vi "cursor window logic V3.vi"(4 "h. offset":dbl, 6 "CursIdx":i32, 7 "cursor window action":T3=enum."check", 8 "window":dbl=nan, 9 "center":dbl=nan, 10 "cursor window in":refnum<vi>, 11 "cursor window init":T2={"left"=2378.60310421286, "right "=2421.6740576496672, "center"=2421.6740576496672, "window"=2421.6740576496672, "cursors"=[], "relative"=0, "absolute"=0, "fixed vertical offset"=2421.6740576496672, "vertical offset"=2421.6740576496672, "skew"=2421.6740576496672, "default window frac"=2421.6740576496672, "kind"=enum."skewed", "skew.left"=2421.6740576496672, "skew.right"=2421.6740576496672, "Plot ref"=refnum, "wing order"=enum."back"}) -> (2 "cursor window out":refnum<vi>, 3 "cursor window out":T2={"left"=2378.60310421286, "right "=2421.6740576496672, "center"=2421.6740576496672, "window"=2421.6740576496672, "cursors"=[], "relative"=0, "absolute"=0, "fixed vertical offset"=2421.6740576496672, "vertical offset"=2421.6740576496672, "skew"=2421.6740576496672, "default window frac"=2421.6740576496672, "kind"=enum."skewed", "skew.left"=2421.6740576496672, "skew.right"=2421.6740576496672, "Plot ref"=refnum, "wing order"=enum."back"})   [LabVIEW 2020]
uses:
  cursor window action.ctl
  cursor winow.ctl
  comparison control.ctl
  cursor window state.ctl
  stack action -- control.ctl
  cursor action.ctl
  2Dwindow.ctl
  range multiplier action.ctl
  cursor sate.ctl
  Q - not nan -- real.vi
  Q - not nan -- integer.vi
panel:
  out "selector":T1
  out "result":bool
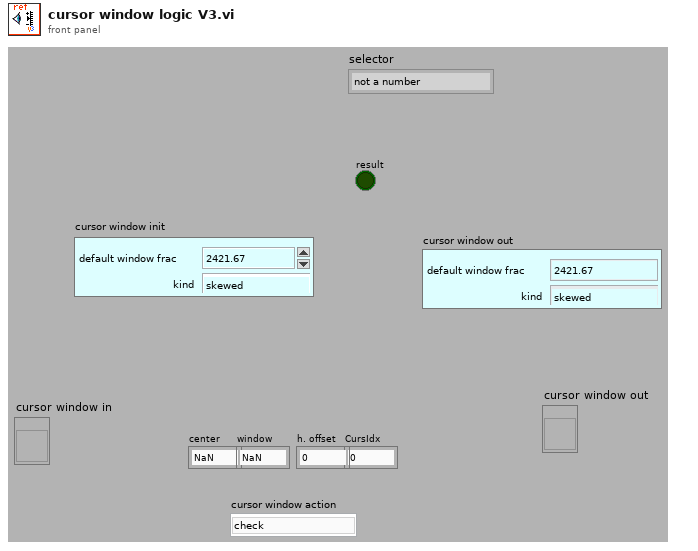
[diagram p1: front panel]
types:
  T1 = typedef "comparison control.ctl" = enum16{"not a number", "above", "in range", "below"}
  T2 = typedef "cursor winow.ctl" = cluster{"left":dbl, "right ":dbl, "center":dbl, "window":dbl, "cursors":i32[], "relative":i32, "absolute":i32, "fixed vertical offset":dbl, "vertical offset":dbl, "skew":dbl, "default window frac":dbl, "kind":enum16{"symmetric", "skewed", "fancy"}, "skew.left":dbl, "skew.right":dbl, "Plot ref":refnum<vi>, "wing order":enum16{"forw", "back"}}
  T3 = typedef "cursor window action.ctl" = enum16{"balance", "h. offset change", "cursor moves", "change center", "change window", "init", "check", "reset", "set y to middle", "idle", "-write all Y", "-write left.X", "-write center.X", "-write right.X", "-write all X", "-change center", "-change window", "-change skew", "-read cursor 2", "-read cursor 1", "-read cursor 0", "-read all cursors", "-reset", "-read plot scale", "-set y to middle", "-Q: center.Y is visible", "-Q: window is visible", "-parse center.Y", "-right left from center", "-left move", "-right move", "-set center.Y", "-empty", "-set cursors to default", "-check", "-write center.Y", "-copy cursor 1", "-copy cursor 0", "-copy cursor 2", "move right", "move left", "shrink", "broaden", "skew up", "skew down", "-write plot scale", "zoom X", "change cen&win", "zoom to all data", "color--red", "color--green", "color--yellow", "read", "zoom out", "zoom in", "slide right", "slide left", "set range aspect ratio to 1"}
  T4 = typedef "cursor window state.ctl" = cluster{"right.Y":dbl, "right.X":dbl, "left.X":dbl, "left.Y":dbl, "center.X":dbl, "center.Y":dbl, "scale.x.max":dbl, "scale.x.min":dbl, "scale.y.range":dbl, "scale.y.min":dbl, "scale.x.range":dbl, "scale.y.max":dbl, "skew":dbl, "cursor":i32, "scale.x.center":dbl, "scale.x.halfwidth":dbl, "scale.y.center":dbl, "scale.y.halfwidth":dbl}
  T5 = typedef "stack action -- control.ctl" = enum16{"push", "pop", "check", "init"}
  T6 = cluster{"center":dbl, "window":dbl, "h.offset":dbl, "cursor window":T2}
  T7 = cluster{"right.Y":dbl, "right.X":dbl, "left.X":dbl, "left.Y":dbl, "center.X":dbl, "center.Y":dbl, "scale.x.max":dbl, "scale.x.min":dbl, "scale.y.range":dbl, "scale.y.min":dbl, "scale.x.range":dbl, "scale.y.max":dbl, "skew":dbl, "cursor":i32, "scale.x.center":dbl, "scale.x.halfwidth":dbl, "scale.y.center":dbl, "scale.y.halfwidth":dbl}
  T8 = cluster{"left":dbl, "right ":dbl, "center":dbl, "window":dbl, "cursors":i32[], "relative":i32, "absolute":i32, "fixed vertical offset":dbl, "vertical offset":dbl, "skew":dbl, "default window frac":dbl, "kind":enum16{"symmetric", "skewed", "fancy"}, "skew.left":dbl, "skew.right":dbl, "Plot ref":refnum<vi>, "wing order":enum16{"forw", "back"}}
  T9 = typedef "cursor action.ctl" = enum16{"range", "read", "write", "check", "zoom out", "smart zoom out", "zoom to aspect ratio 1", "zoom to win", "zoom out 20%", "zoom in 20%", "-empty", "smart zoom out&aspect", "move range left 20%", "move range right 20%", "move range up 20%", "move range down 20%", "zoom to X win", "zoom to Y win", "zoom out X", "zoom out Y", "zoom in X", "zoom in Y", "check plot scale"}
  T10 = typedef "2Dwindow.ctl" = cluster{"window y":dbl, "center x":dbl, "center y":dbl, "window x":dbl}
  T11 = typedef "range multiplier action.ctl" = enum16{"shift", "zoom", "check"}
  T12 = typedef "2Dwindow-bounds.ctl" = cluster{"min y":dbl, "max x":dbl, "min x":dbl, "max y":dbl}
  T13 = typedef "cursor sate.ctl" = enum16{"normal", "alert", "fuzzy", "interesting", "boring", "colored"}
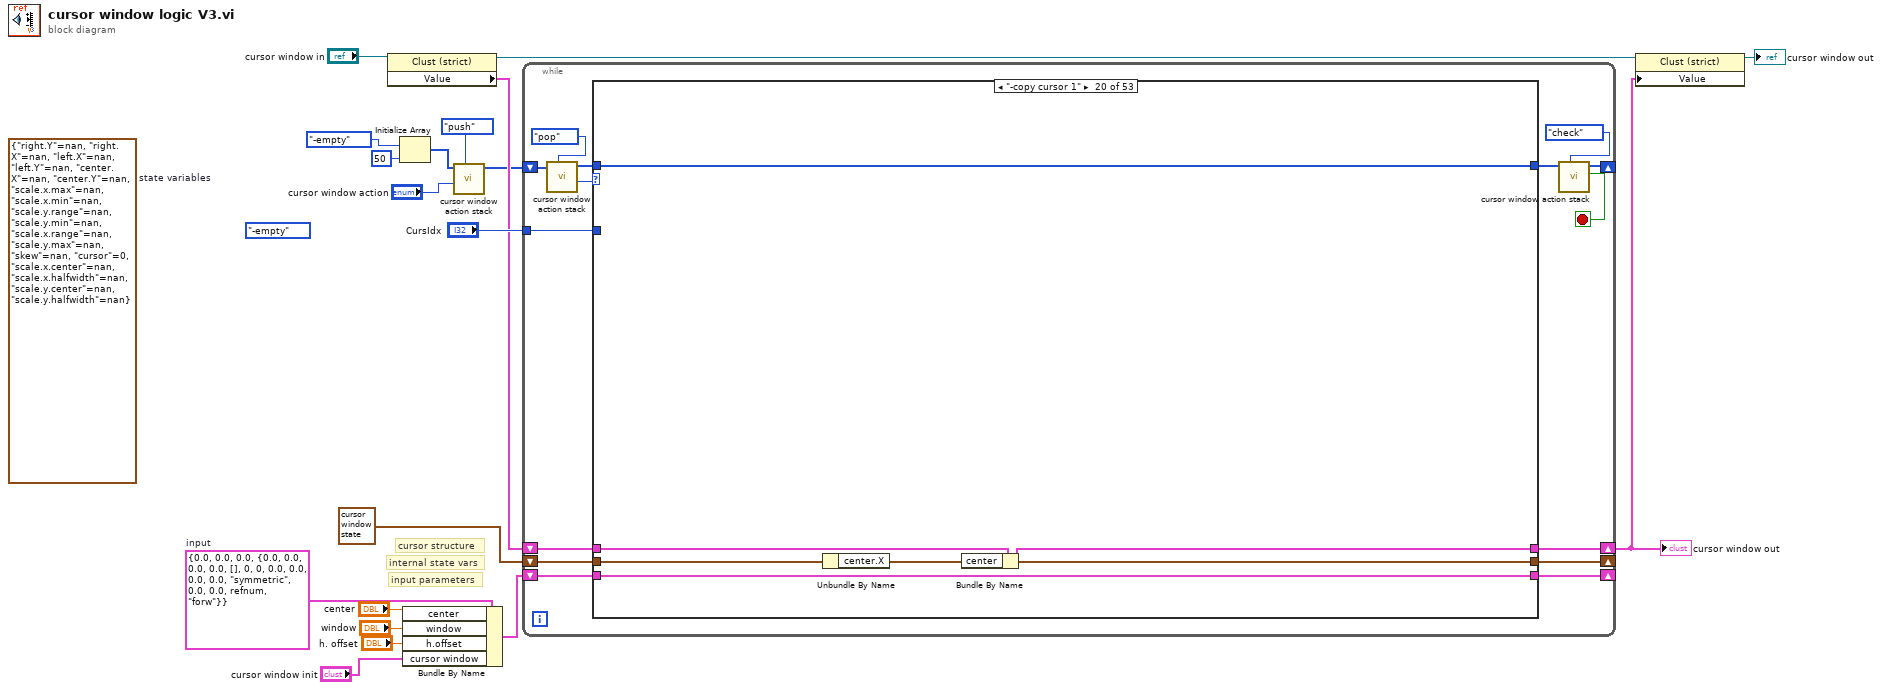
[diagram p0: block diagram]
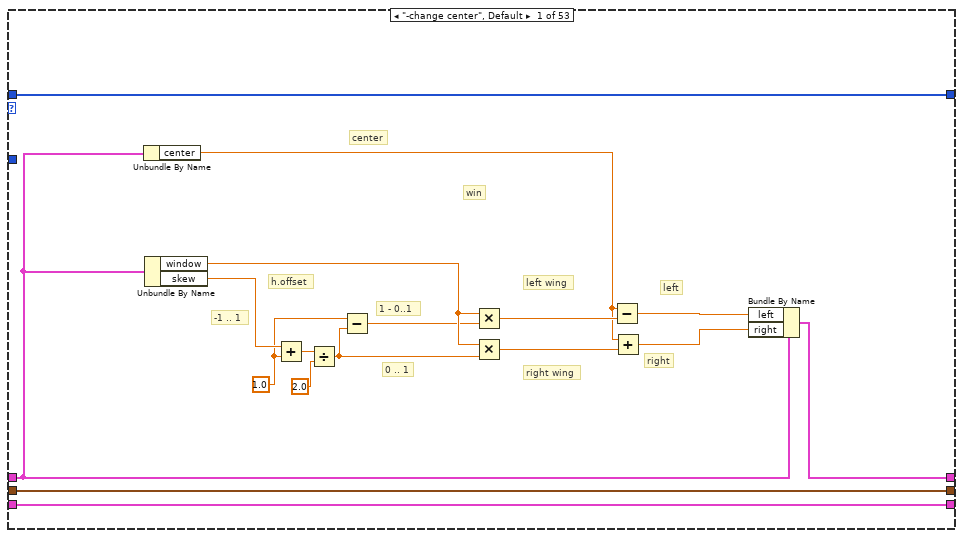
[diagram p2: hidden frame]
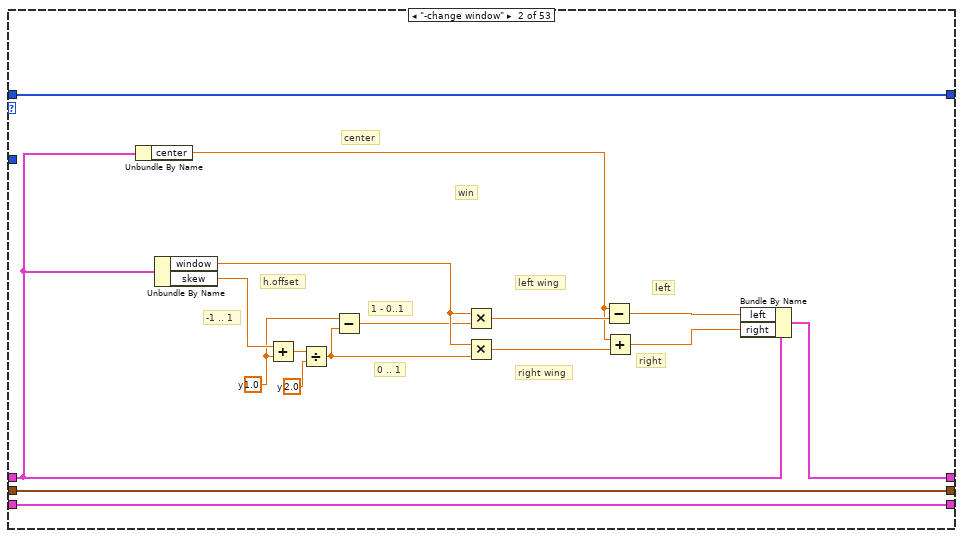
[diagram p3: hidden frame]
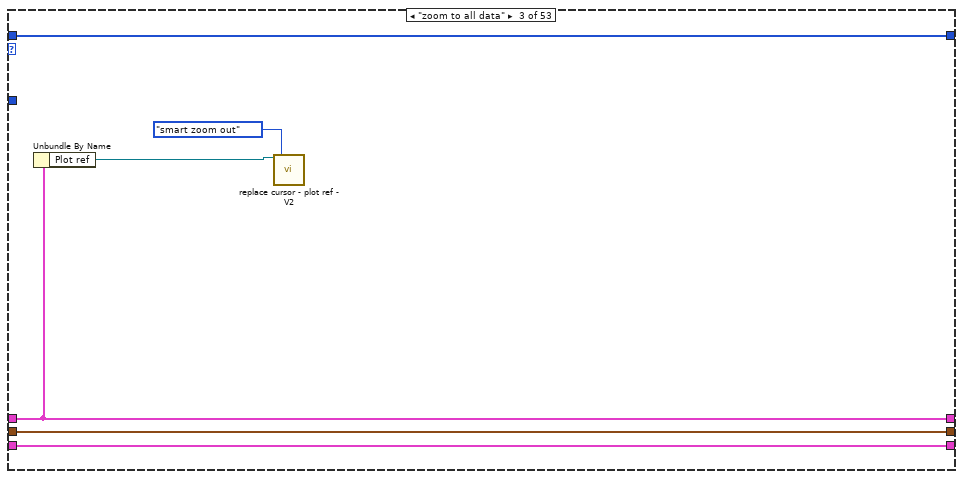
[diagram p4: hidden frame]
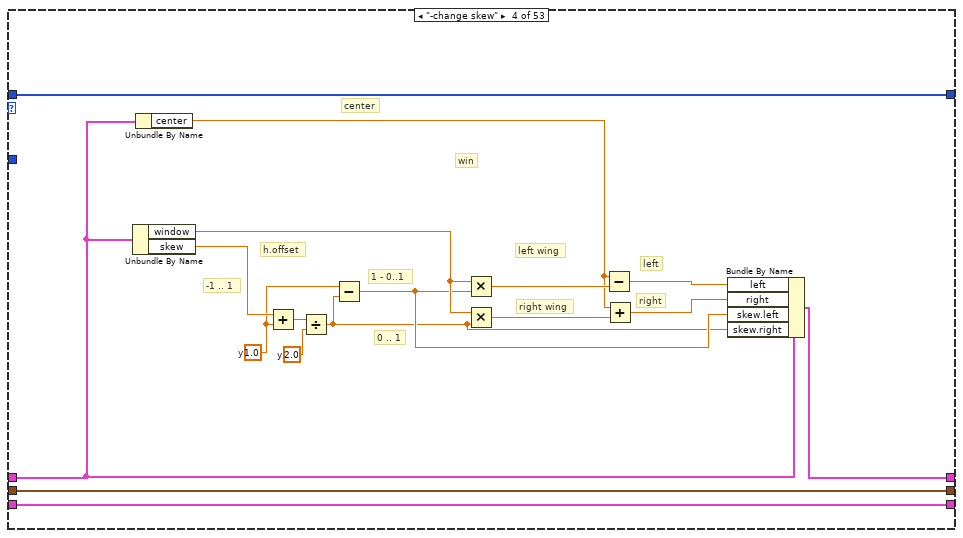
[diagram p5: hidden frame]
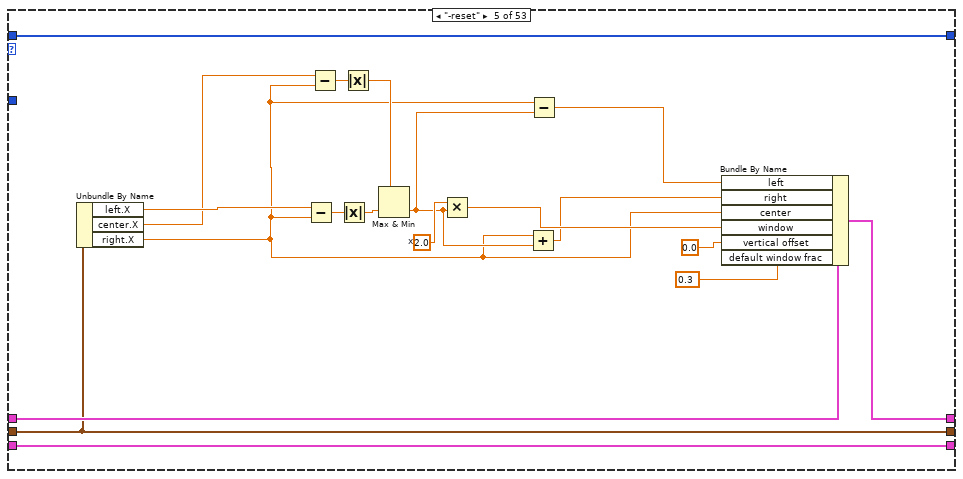
[diagram p6: hidden frame]
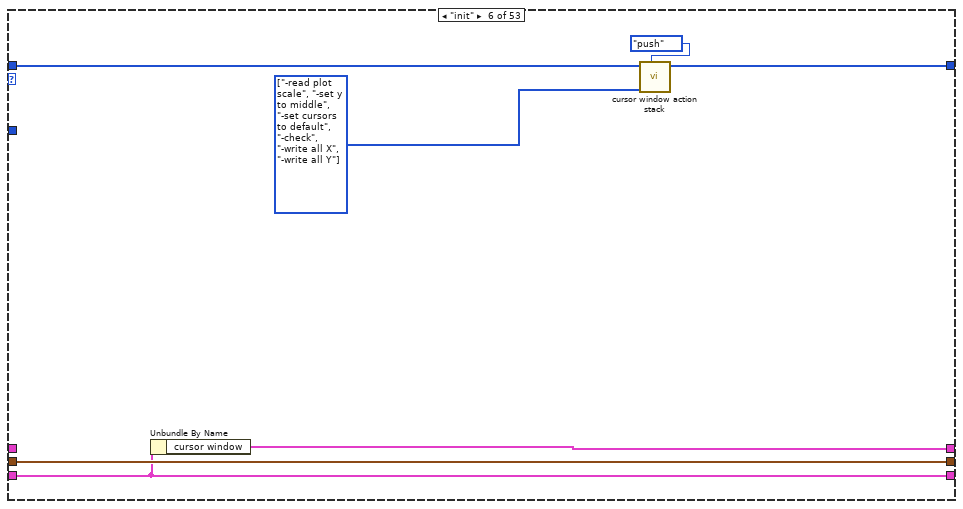
[diagram p7: hidden frame]
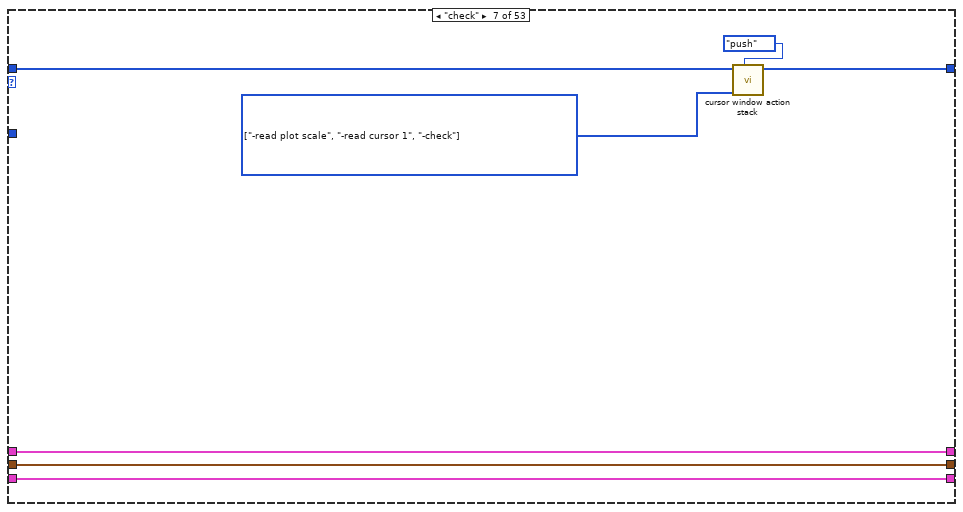
[diagram p8: hidden frame]
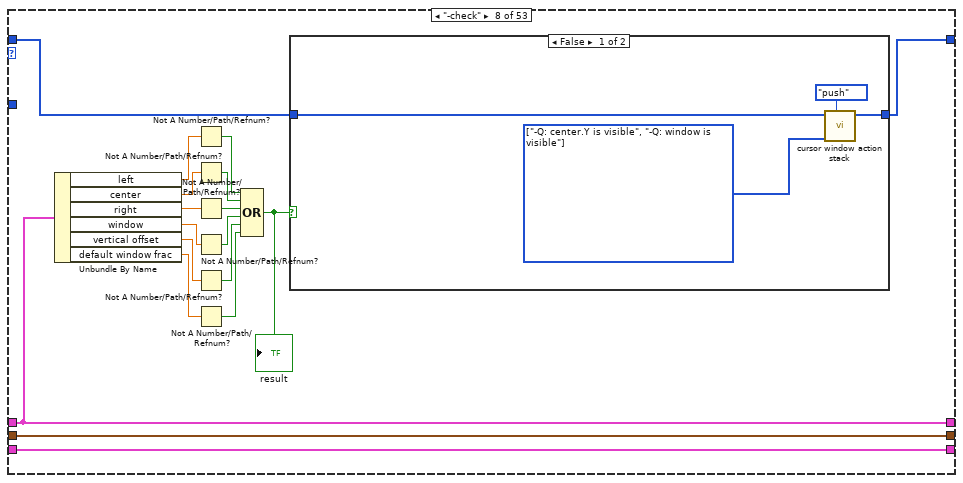
[diagram p9: hidden frame]
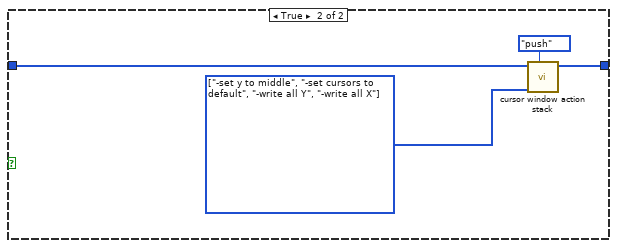
[diagram p10: hidden frame]
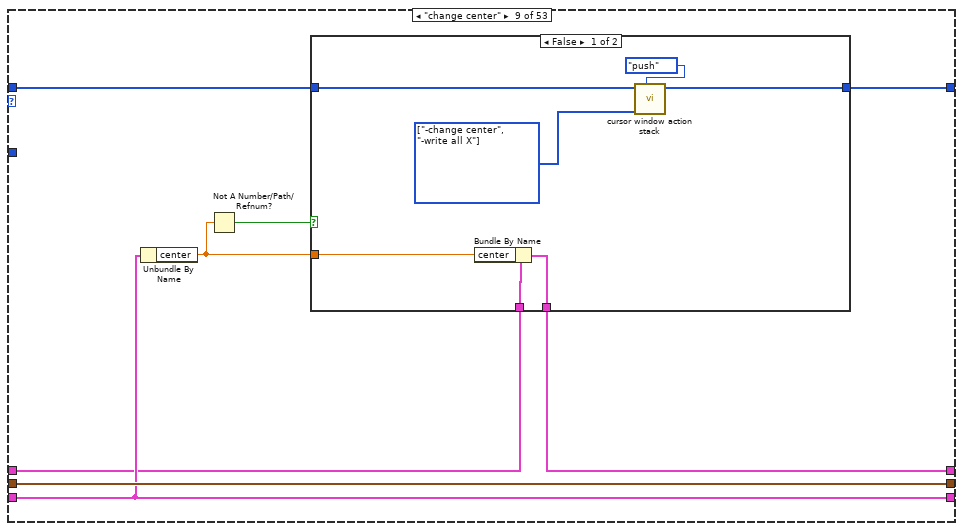
[diagram p11: hidden frame]
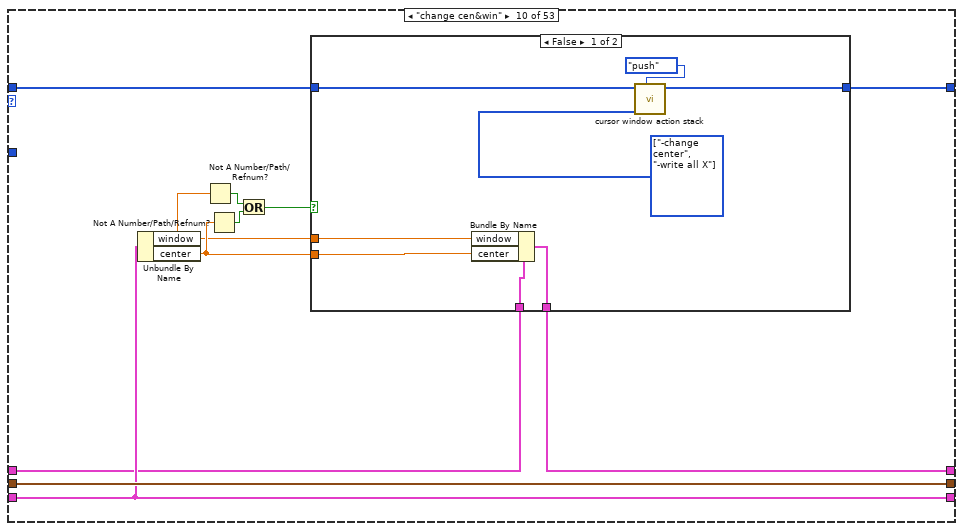
[diagram p13: hidden frame]
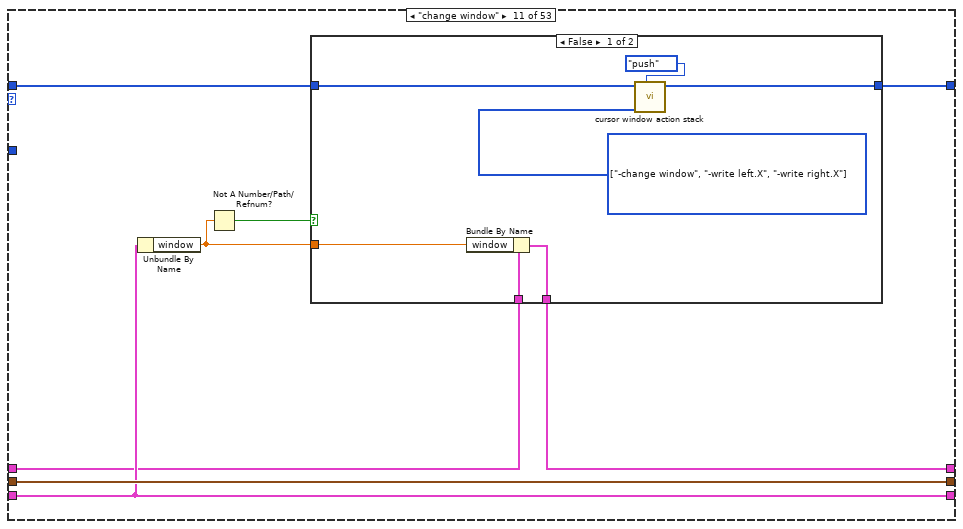
[diagram p15: hidden frame]
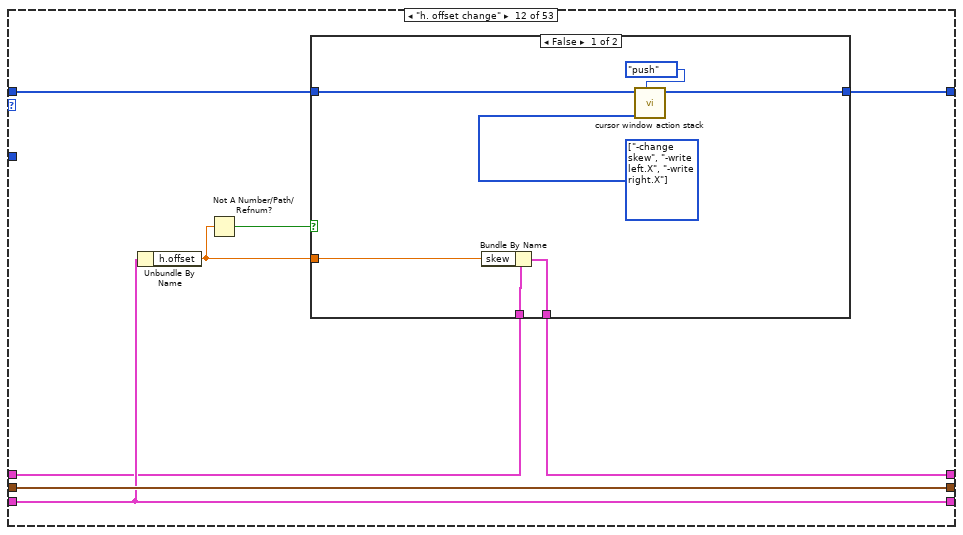
[diagram p17: hidden frame]
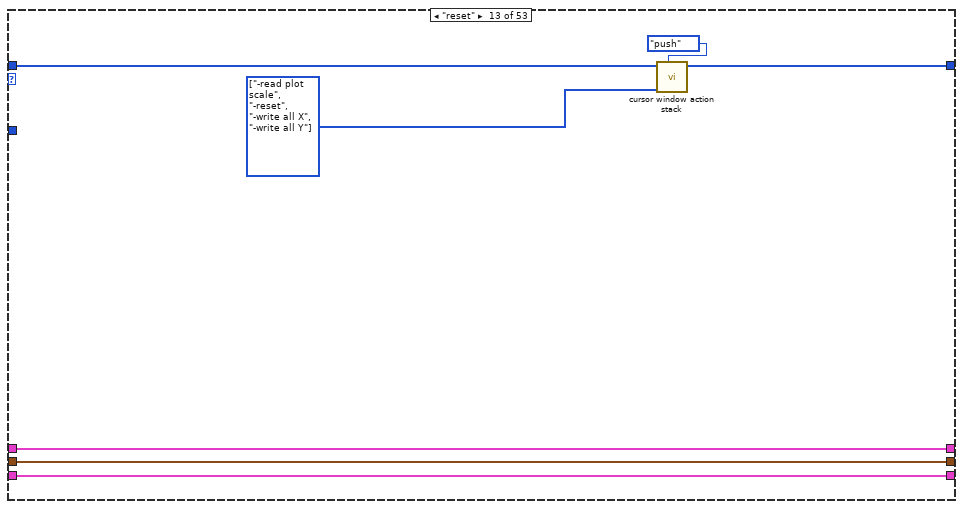
[diagram p19: hidden frame]
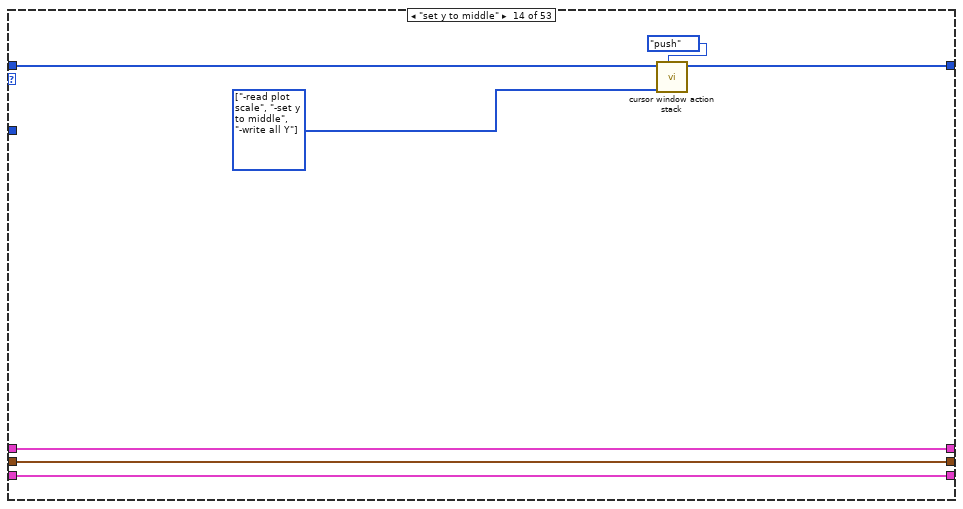
[diagram p20: hidden frame]
diagram:
  (unwired) cursor_window_action."-empty" ("cursor window action")
  w18 = T6 {"center"=0.0, "window"=0.0, "h.offset"=0.0, "cursor window"={"left"=0.0, "right "=0.0, "center"=0.0, "window"=0.0, "cursors"=[], "relative"=0, "absolute"=0, "fixed vertical offset"=0.0, "vertical offset"=0.0, "skew"=0.0, "default window frac"=0.0, "kind"=enum."symmetric", "skew.left"=0.0, "skew.right"=0.0, "Plot ref"=refnum, "wing order"=enum."forw"}}  # input
  (unwired) T7 {"right.Y"=nan, "right.X"=nan, "left.X"=nan, "left.Y"=nan, "center.X"=nan, "center.Y"=nan, "scale.x.max"=nan, "scale.x.min"=nan, "scale.y.range"=nan, "scale.y.min"=nan, "scale.x.range"=nan, "scale.y.max"=nan, "skew"=nan, "cursor"=0, "scale.x.center"=nan, "scale.x.halfwidth"=nan, "scale.y.center"=nan, "scale.y.halfwidth"=nan}  # state variables
  # "input parameters"
  # "internal state vars"
  # "cursor structure"
  n1 = property class="Clust (strict)"(reference="cursor window in") -> (reference out=w19:refnum<vi>, "Value"=w12:T8)  [unwired: 1 in, 1 out]
  n2 = Initialize Array(cursor_window_action."-empty" ("cursor window action"), 50 ("dimension size")) -> (w5:T3[])
  n3 = Bundle By Name(cluster=w18, "center"="center", "window"="window", "h.offset"="h. offset", "cursor window"="cursor window init") -> (w14:T6)
  n4 = call "cursor window action stack.vi"("stack action"=stack_action_--_control."push", "cursor window action"="cursor window action", "command stack"=w5) -> ("command stack out"=w4:T3[])  [unwired: 6 in, 2 out]
  n5 = while {
    shift-right: [w27] -> _
    shift-left: w4 -> [w33]
    shift-right: [w20] -> w11
    shift-left: w12 -> [w34]
    shift-right: [w24] -> _
    shift-left: w14 -> [w25]
    shift-right: [w22] -> _
    shift-left: T4 {"right.Y"=nan, "right.X"=nan, "left.X"=nan, "left.Y"=nan, "center.X"=nan, "center.Y"=nan, "scale.x.max"=nan, "scale.x.min"=nan, "scale.y.range"=nan, "scale.y.min"=nan, "scale.x.range"=nan, "scale.y.max"=nan, "skew"=nan, "cursor"=0, "scale.x.center"=nan, "scale.x.halfwidth"=nan, "scale.y.center"=nan, "scale.y.halfwidth"=nan} ("state variables") -> [w23]
    tunnel: "CursIdx" -> [w21]
    stop <- w26 stop-if-true
    n6 = call "cursor window action stack.vi"("stack action"=stack_action_--_control."pop", "command stack"=w33) -> ("cursor window action out"=w32:T3, "command stack out"=w30:T3[])  [unwired: 7 in, 1 out]
    n7 = case shown="\"-copy cursor 1\"" w32 {
      tunnel: w34 -> [w36 w53 w71 w78 w100 _ w118 w128 w152 w173 w190 w207 w223 w230 w247 w281 w316 w355 w387 w391 w398 w417 w431 w457 w472 w478 w484 w490 w496 w502 w509 w533 w539 w559 w565 w578 w599 w638 w672 w712 w733 w753 w773 w794 w808 w825 w844 w857 w866 w889 w893 w906 w920]
      tunnel: [w40 w57 w74 w82 w99 w112 w121 w125 w157 w177 w195 w212 w226 w233 w244 w278 w318 w356 w388 w389 w407 w423 w442 w458 w473 w479 w485 w491 w497 w503 w507 w534 w547 w560 w574 w582 w603 w636 w674 w729 w749 w769 w789 w807 w822 w839 w853 w865 w887 w891 w905 w919 w933] -> w28
      tunnel: w30 -> [w40 w57 w74 w82 w99 w113 w122 w126 w156 w176 w194 w211 w227 w234 w244 w278 w318 w343 w388 w389 w407 w423 w442 w458 w473 w479 w485 w491 w497 w503 w508 w535 w548 w561 w575 w583 w604 w636 w675 w729 w749 w769 w789 w807 w822 w839 w853 w865 w887 w891 w905 w919 w933]
      tunnel: w25 -> [w37 w54 w72 w79 w98 w116 w119 w129 w155 w175 w193 w210 w229 w236 w246 w280 w317 w348 w385 w392 w406 w422 w445 w459 w474 w480 w486 w492 w498 w504 w515 w529 w545 w555 w572 w579 w600 w654 w679 w714 w735 w755 w775 w796 w814 w832 w846 w859 w868 w890 w895 w909 w923]
      tunnel: [w37 w54 w72 w79 w98 w116 w119 w129 w155 w175 w193 w210 w229 w236 w246 w280 w317 w348 w385 w392 w406 w422 w445 w459 w474 w480 w486 w492 w498 w504 w515 w529 w545 w555 w572 w579 w600 w654 w679 w714 w735 w755 w775 w796 w814 w832 w846 w859 w868 w890 w895 w909 w923] -> w24
      tunnel: w23 -> [w39 w56 w73 w81 w97 w117 w120 w130 w158 w178 w196 w213 w228 w235 w245 w279 w322 w349 w386 w394 w403 w421 w444 w456 w471 w477 w483 w489 w495 w501 w511 w530 w546 w556 w573 w580 w601 w642 w678 w715 w736 w756 w776 w793 w815 w833 w847 w856 w876 w888 w899 w913 w927]
      tunnel: [w39 w56 w73 w81 w97 w117 w120 w130 w158 w178 w196 w213 w228 w235 w245 w279 w321 w349 w386 w394 w402 w421 w443 w456 w471 w477 w483 w489 w495 w501 w510 w530 w546 w556 w573 w580 w601 w645 w678 w715 w736 w756 w776 w793 w815 w833 w847 w856 w875 w888 w898 w912 w926] -> w22
      tunnel: w21 -> [_ _ _ _ _ _ _ _ _ _ _ _ _ _ _ _ _ w346 _ _ _ _ _ _ _ _ _ _ _ _ _ _ _ _ _ _ _ _ _ _ _ _ _ _ _ _ _ _ _ _ _ _ _]
      tunnel: [w35 w52 w71 w77 w93 w111 w118 w128 w151 w172 w189 w206 w223 w230 w237 w271 w316 w347 w387 w390 w397 w413 w431 w457 w472 w478 w484 w490 w496 w502 w509 w532 w538 w558 w564 w581 w602 w634 w671 w712 w733 w753 w773 w794 w808 w825 w844 w857 w866 w889 w893 w906 w920] -> w20
      frame "-change center", Default {
        w45 = 1.0 ("y")
        # "1 - 0..1"
        # "right"
        # "left"
        # "win"
        # "h.offset"
        # "center"
        # "left wing"
        # "right wing"
        # "0 .. 1"
        # "-1 .. 1"
        n8 = Unbundle By Name(w36) -> ("center"=w38:dbl)
        n9 = Unbundle By Name(w36) -> ("window"=w50:dbl, "skew"=w51:dbl)
        n10 = Add(x=w51, y=w45) -> (x+y=w46:dbl)
        n11 = Divide(x=w46, y=2.0) -> (x/y=w42:dbl)
        n12 = Subtract(x=w45, y=w42) -> (x-y=w41:dbl)
        n13 = Multiply(x=w50, y=w41) -> (x*y=w44:dbl)
        n14 = Multiply(x=w50, y=w42) -> (x*y=w43:dbl)
        n15 = Subtract(x=w38, y=w44) -> (x-y=w49:dbl)
        n16 = Add(x=w38, y=w43) -> (x+y=w48:dbl)
        n17 = Bundle By Name(cluster=w36, "left"=w49, "right"=w48) -> (w35:T2)
      }
      frame "-change window" {
        w62 = 1.0  # y
        w64 = 2.0  # y
        # "1 - 0..1"
        # "right"
        # "left"
        # "win"
        # "h.offset"
        # "center"
        # "left wing"
        # "right wing"
        # "0 .. 1"
        # "-1 .. 1"
        n18 = Unbundle By Name(w53) -> ("center"=w55:dbl)
        n19 = Unbundle By Name(w53) -> ("window"=w67:dbl, "skew"=w68:dbl)
        n20 = Add(x=w68, y=w62) -> (x+y=w63:dbl)
        n21 = Divide(x=w63, y=w64) -> (x/y=w59:dbl)
        n22 = Subtract(x=w62, y=w59) -> (x-y=w58:dbl)
        n23 = Multiply(x=w67, y=w58) -> (x*y=w61:dbl)
        n24 = Multiply(x=w67, y=w59) -> (x*y=w60:dbl)
        n25 = Subtract(x=w55, y=w61) -> (x-y=w66:dbl)
        n26 = Add(x=w55, y=w60) -> (x+y=w65:dbl)
        n27 = Bundle By Name(cluster=w53, "left"=w66, "right"=w65) -> (w52:T2)
      }
      frame "zoom to all data" {
        n28 = Unbundle By Name(w71) -> ("Plot ref"=w70:refnum<vi>)
        n29 = call "replace cursor - plot ref - V2.vi"("Plot ref in"=w70, "cursor action"=cursor_action."smart zoom out") -> ()  [unwired: 14 in, 4 out]
      }
      frame "-change skew" {
        w85 = 1.0  # y
        w87 = 2.0  # y
        # "1 - 0..1"
        # "right"
        # "left"
        # "win"
        # "h.offset"
        # "center"
        # "left wing"
        # "right wing"
        # "0 .. 1"
        # "-1 .. 1"
        n30 = Unbundle By Name(w78) -> ("window"=w90:dbl, "skew"=w91:dbl)
        n31 = Unbundle By Name(w78) -> ("center"=w80:dbl)
        n32 = Add(x=w91, y=w85) -> (x+y=w86:dbl)
        n33 = Divide(x=w86, y=w87) -> (x/y=w75:dbl)
        n34 = Subtract(x=w85, y=w75) -> (x-y=w76:dbl)
        n35 = Multiply(x=w90, y=w76) -> (x*y=w84:dbl)
        n36 = Multiply(x=w90, y=w75) -> (x*y=w83:dbl)
        n37 = Subtract(x=w80, y=w84) -> (x-y=w89:dbl)
        n38 = Add(x=w80, y=w83) -> (x+y=w88:dbl)
        n39 = Bundle By Name(cluster=w78, "left"=w89, "right"=w88, "skew.left"=w76, "skew.right"=w75) -> (w77:T2)
      }
      frame "-reset" {
        w106 = 2.0  # x
        n40 = Unbundle By Name(w97) -> ("left.X"=w96:dbl, "center.X"=w94:dbl, "right.X"=w95:dbl)
        n41 = Subtract(x=w96, y=w95) -> (x-y=w109:dbl)
        n42 = Subtract(x=w94, y=w95) -> (x-y=w110:dbl)
        n43 = Absolute Value(x=w109) -> (abs(x)=w107:dbl)
        n44 = Absolute Value(x=w110) -> (abs(x)=w108:dbl)
        n45 = Max & Min(x=w108, y=w107) -> (min(x,y)=w104:dbl)  [unwired: 1 out]
        n46 = Multiply(x=w106, y=w104) -> (x*y=w105:dbl)
        n47 = Add(x=w95, y=w104) -> (x+y=w102:dbl)
        n48 = Subtract(x=w95, y=w104) -> (x-y=w103:dbl)
        n49 = Bundle By Name(cluster=w100, "left"=w103, "right"=w102, "center"=w95, "window"=w105, "vertical offset"=0.0, "default window frac"=0.3) -> (w93:T2)
      }
      frame "init" {
        w114 = T3[] [enum."-read plot scale", enum."-set y to middle", enum."-set cursors to default", enum."-check", enum."-write all X", enum."-write all Y"] items=["balance", "h. offset change", "cursor moves", "change center", "change window", "init", "check", "reset", "set y to middle", "idle", "-write all Y", "-write left.X", "-write center.X", "-write right.X", "-write all X", "-change center", "-change window", "-change skew", "-read cursor 2", "-read cursor 1", "-read cursor 0", "-read all cursors", "-reset", "-read plot scale", "-set y to middle", "-Q: center.Y is visible", "-Q: window is visible", "-parse center.Y", "-right left from center", "-left move", "-right move", "-set center.Y", "-empty", "-set cursors to default", "-check", "-write center.Y", "-copy cursor 1", "-copy cursor 0", "-copy cursor 2", "move right", "move left", "shrink", "broaden", "skew up", "skew down", "-write plot scale", "zoom X", "change cen&win", "zoom to all data", "color--red", "color--green", "color--yellow", "read", "zoom out", "zoom in", "slide right", "slide left", "set range aspect ratio to 1"]
        n50 = Unbundle By Name(w116) -> ("cursor window"=w111:T2)
        n51 = call "cursor window action stack.vi"("stack action"=stack_action_--_control."push", "action list"=w114, "command stack"=w113) -> ("command stack out"=w112:T3[])  [unwired: 6 in, 2 out]
      }
      frame "check" {
        w123 = T3[] [enum."-read plot scale", enum."-read cursor 1", enum."-check"] items=["balance", "h. offset change", "cursor moves", "change center", "change window", "init", "check", "reset", "set y to middle", "idle", "-write all Y", "-write left.X", "-write center.X", "-write right.X", "-write all X", "-change center", "-change window", "-change skew", "-read cursor 2", "-read cursor 1", "-read cursor 0", "-read all cursors", "-reset", "-read plot scale", "-set y to middle", "-Q: center.Y is visible", "-Q: window is visible", "-parse center.Y", "-right left from center", "-left move", "-right move", "-set center.Y", "-empty", "-set cursors to default", "-check", "-write center.Y", "-copy cursor 1", "-copy cursor 0", "-copy cursor 2", "move right", "move left", "shrink", "broaden", "skew up", "skew down", "-write plot scale", "zoom X", "change cen&win", "zoom to all data", "color--red", "color--green", "color--yellow", "read", "zoom out", "zoom in", "slide right", "slide left", "set range aspect ratio to 1"]
        n52 = call "cursor window action stack.vi"("stack action"=stack_action_--_control."push", "action list"=w123, "command stack"=w122) -> ("command stack out"=w121:T3[])  [unwired: 6 in, 2 out]
      }
      frame "-check" {
        n53 = Unbundle By Name(w128) -> ("left"=w140:dbl, "center"=w139:dbl, "right"=w141:dbl, "window"=w142:dbl, "vertical offset"=w134:dbl, "default window frac"=w133:dbl)
        n54 = Not A Number/Path/Refnum?(number/path/refnum=w140) -> (NaN/Path/Refnum?=w138:bool)
        n55 = Not A Number/Path/Refnum?(number/path/refnum=w139) -> (NaN/Path/Refnum?=w137:bool)
        n56 = Not A Number/Path/Refnum?(number/path/refnum=w141) -> (NaN/Path/Refnum?=w136:bool)
        n57 = Not A Number/Path/Refnum?(number/path/refnum=w142) -> (NaN/Path/Refnum?=w135:bool)
        n58 = Not A Number/Path/Refnum?(number/path/refnum=w134) -> (NaN/Path/Refnum?=w131:bool)
        n59 = Not A Number/Path/Refnum?(number/path/refnum=w133) -> (NaN/Path/Refnum?=w132:bool)
        n60 = Compound Arithmetic op=OR(w138, w137, w136, w135, w131, w132) -> (w127:bool)
        "result" <- w127
        n61 = case shown="False" w127 {
          tunnel: w126 -> [w144 w148]
          tunnel: [w143 w147] -> w125
          frame False {
            w145 = T3[] [enum."-Q: center.Y is visible", enum."-Q: window is visible"] items=["balance", "h. offset change", "cursor moves", "change center", "change window", "init", "check", "reset", "set y to middle", "idle", "-write all Y", "-write left.X", "-write center.X", "-write right.X", "-write all X", "-change center", "-change window", "-change skew", "-read cursor 2", "-read cursor 1", "-read cursor 0", "-read all cursors", "-reset", "-read plot scale", "-set y to middle", "-Q: center.Y is visible", "-Q: window is visible", "-parse center.Y", "-right left from center", "-left move", "-right move", "-set center.Y", "-empty", "-set cursors to default", "-check", "-write center.Y", "-copy cursor 1", "-copy cursor 0", "-copy cursor 2", "move right", "move left", "shrink", "broaden", "skew up", "skew down", "-write plot scale", "zoom X", "change cen&win", "zoom to all data", "color--red", "color--green", "color--yellow", "read", "zoom out", "zoom in", "slide right", "slide left", "set range aspect ratio to 1"]
            n62 = call "cursor window action stack.vi"("stack action"=stack_action_--_control."push", "action list"=w145, "command stack"=w144) -> ("command stack out"=w143:T3[])  [unwired: 6 in, 2 out]
          }
          frame True {
            w149 = T3[] [enum."-set y to middle", enum."-set cursors to default", enum."-write all Y", enum."-write all X"] items=["balance", "h. offset change", "cursor moves", "change center", "change window", "init", "check", "reset", "set y to middle", "idle", "-write all Y", "-write left.X", "-write center.X", "-write right.X", "-write all X", "-change center", "-change window", "-change skew", "-read cursor 2", "-read cursor 1", "-read cursor 0", "-read all cursors", "-reset", "-read plot scale", "-set y to middle", "-Q: center.Y is visible", "-Q: window is visible", "-parse center.Y", "-right left from center", "-left move", "-right move", "-set center.Y", "-empty", "-set cursors to default", "-check", "-write center.Y", "-copy cursor 1", "-copy cursor 0", "-copy cursor 2", "move right", "move left", "shrink", "broaden", "skew up", "skew down", "-write plot scale", "zoom X", "change cen&win", "zoom to all data", "color--red", "color--green", "color--yellow", "read", "zoom out", "zoom in", "slide right", "slide left", "set range aspect ratio to 1"]
            n63 = call "cursor window action stack.vi"("stack action"=stack_action_--_control."push", "action list"=w149, "command stack"=w148) -> ("command stack out"=w147:T3[])  [unwired: 6 in, 2 out]
          }
        }
      }
      frame "change center" {
        n64 = Unbundle By Name(w155) -> ("center"=w153:dbl)
        n65 = Not A Number/Path/Refnum?(number/path/refnum=w153) -> (NaN/Path/Refnum?=w154:bool)
        n66 = case shown="False" w154 {
          tunnel: [w165 w166] -> w157
          tunnel: w156 -> [w164 w166]
          tunnel: w152 -> [w161 w167]
          tunnel: w153 -> [w160 _]
          tunnel: [w159 w167] -> w151
          frame False {
            w162 = T3[] [enum."-change center", enum."-write all X"] items=["balance", "h. offset change", "cursor moves", "change center", "change window", "init", "check", "reset", "set y to middle", "idle", "-write all Y", "-write left.X", "-write center.X", "-write right.X", "-write all X", "-change center", "-change window", "-change skew", "-read cursor 2", "-read cursor 1", "-read cursor 0", "-read all cursors", "-reset", "-read plot scale", "-set y to middle", "-Q: center.Y is visible", "-Q: window is visible", "-parse center.Y", "-right left from center", "-left move", "-right move", "-set center.Y", "-empty", "-set cursors to default", "-check", "-write center.Y", "-copy cursor 1", "-copy cursor 0", "-copy cursor 2", "move right", "move left", "shrink", "broaden", "skew up", "skew down", "-write plot scale", "zoom X", "change cen&win", "zoom to all data", "color--red", "color--green", "color--yellow", "read", "zoom out", "zoom in", "slide right", "slide left", "set range aspect ratio to 1"]
            n67 = Bundle By Name(cluster=w161, "center"=w160) -> (w159:T2)
            n68 = call "cursor window action stack.vi"("stack action"=stack_action_--_control."push", "action list"=w162, "command stack"=w164) -> ("command stack out"=w165:T3[])  [unwired: 6 in, 2 out]
          }
          frame True {
          }
        }
      }
      frame "change cen&win" {
        n69 = Unbundle By Name(w175) -> ("window"=w168:dbl, "center"=w174:dbl)
        n70 = Not A Number/Path/Refnum?(number/path/refnum=w168) -> (NaN/Path/Refnum?=w171:bool)
        n71 = Not A Number/Path/Refnum?(number/path/refnum=w174) -> (NaN/Path/Refnum?=w170:bool)
        n72 = Or(x=w171, y=w170) -> (x .or. y?=w169:bool)
        n73 = case shown="False" w169 {
          tunnel: [w186 w187] -> w177
          tunnel: w176 -> [w185 w187]
          tunnel: w173 -> [w182 w188]
          tunnel: w174 -> [w181 _]
          tunnel: [w180 w188] -> w172
          tunnel: w168 -> [w179 _]
          frame False {
            w183 = T3[] [enum."-change center", enum."-write all X"] items=["balance", "h. offset change", "cursor moves", "change center", "change window", "init", "check", "reset", "set y to middle", "idle", "-write all Y", "-write left.X", "-write center.X", "-write right.X", "-write all X", "-change center", "-change window", "-change skew", "-read cursor 2", "-read cursor 1", "-read cursor 0", "-read all cursors", "-reset", "-read plot scale", "-set y to middle", "-Q: center.Y is visible", "-Q: window is visible", "-parse center.Y", "-right left from center", "-left move", "-right move", "-set center.Y", "-empty", "-set cursors to default", "-check", "-write center.Y", "-copy cursor 1", "-copy cursor 0", "-copy cursor 2", "move right", "move left", "shrink", "broaden", "skew up", "skew down", "-write plot scale", "zoom X", "change cen&win", "zoom to all data", "color--red", "color--green", "color--yellow", "read", "zoom out", "zoom in", "slide right", "slide left", "set range aspect ratio to 1"]
            n74 = Bundle By Name(cluster=w182, "window"=w179, "center"=w181) -> (w180:T2)
            n75 = call "cursor window action stack.vi"("stack action"=stack_action_--_control."push", "action list"=w183, "command stack"=w185) -> ("command stack out"=w186:T3[])  [unwired: 6 in, 2 out]
          }
          frame True {
          }
        }
      }
      frame "change window" {
        n76 = Unbundle By Name(w193) -> ("window"=w191:dbl)
        n77 = Not A Number/Path/Refnum?(number/path/refnum=w191) -> (NaN/Path/Refnum?=w192:bool)
        n78 = case shown="False" w192 {
          tunnel: [w203 w204] -> w195
          tunnel: w194 -> [w202 w204]
          tunnel: w190 -> [w199 w205]
          tunnel: w191 -> [w198 _]
          tunnel: [w197 w205] -> w189
          frame False {
            w200 = T3[] [enum."-change window", enum."-write left.X", enum."-write right.X"] items=["balance", "h. offset change", "cursor moves", "change center", "change window", "init", "check", "reset", "set y to middle", "idle", "-write all Y", "-write left.X", "-write center.X", "-write right.X", "-write all X", "-change center", "-change window", "-change skew", "-read cursor 2", "-read cursor 1", "-read cursor 0", "-read all cursors", "-reset", "-read plot scale", "-set y to middle", "-Q: center.Y is visible", "-Q: window is visible", "-parse center.Y", "-right left from center", "-left move", "-right move", "-set center.Y", "-empty", "-set cursors to default", "-check", "-write center.Y", "-copy cursor 1", "-copy cursor 0", "-copy cursor 2", "move right", "move left", "shrink", "broaden", "skew up", "skew down", "-write plot scale", "zoom X", "change cen&win", "zoom to all data", "color--red", "color--green", "color--yellow", "read", "zoom out", "zoom in", "slide right", "slide left", "set range aspect ratio to 1"]
            n79 = Bundle By Name(cluster=w199, "window"=w198) -> (w197:T2)
            n80 = call "cursor window action stack.vi"("stack action"=stack_action_--_control."push", "action list"=w200, "command stack"=w202) -> ("command stack out"=w203:T3[])  [unwired: 6 in, 2 out]
          }
          frame True {
          }
        }
      }
      frame "h. offset change" {
        n81 = Unbundle By Name(w210) -> ("h.offset"=w208:dbl)
        n82 = Not A Number/Path/Refnum?(number/path/refnum=w208) -> (NaN/Path/Refnum?=w209:bool)
        n83 = case shown="False" w209 {
          tunnel: [w220 w221] -> w212
          tunnel: w211 -> [w219 w221]
          tunnel: w207 -> [w216 w222]
          tunnel: w208 -> [w215 _]
          tunnel: [w214 w222] -> w206
          frame False {
            w217 = T3[] [enum."-change skew", enum."-write left.X", enum."-write right.X"] items=["balance", "h. offset change", "cursor moves", "change center", "change window", "init", "check", "reset", "set y to middle", "idle", "-write all Y", "-write left.X", "-write center.X", "-write right.X", "-write all X", "-change center", "-change window", "-change skew", "-read cursor 2", "-read cursor 1", "-read cursor 0", "-read all cursors", "-reset", "-read plot scale", "-set y to middle", "-Q: center.Y is visible", "-Q: window is visible", "-parse center.Y", "-right left from center", "-left move", "-right move", "-set center.Y", "-empty", "-set cursors to default", "-check", "-write center.Y", "-copy cursor 1", "-copy cursor 0", "-copy cursor 2", "move right", "move left", "shrink", "broaden", "skew up", "skew down", "-write plot scale", "zoom X", "change cen&win", "zoom to all data", "color--red", "color--green", "color--yellow", "read", "zoom out", "zoom in", "slide right", "slide left", "set range aspect ratio to 1"]
            n84 = Bundle By Name(cluster=w216, "skew"=w215) -> (w214:T2)
            n85 = call "cursor window action stack.vi"("stack action"=stack_action_--_control."push", "action list"=w217, "command stack"=w219) -> ("command stack out"=w220:T3[])  [unwired: 6 in, 2 out]
          }
          frame True {
          }
        }
      }
      frame "reset" {
        w224 = T3[] [enum."-read plot scale", enum."-reset", enum."-write all X", enum."-write all Y"] items=["balance", "h. offset change", "cursor moves", "change center", "change window", "init", "check", "reset", "set y to middle", "idle", "-write all Y", "-write left.X", "-write center.X", "-write right.X", "-write all X", "-change center", "-change window", "-change skew", "-read cursor 2", "-read cursor 1", "-read cursor 0", "-read all cursors", "-reset", "-read plot scale", "-set y to middle", "-Q: center.Y is visible", "-Q: window is visible", "-parse center.Y", "-right left from center", "-left move", "-right move", "-set center.Y", "-empty", "-set cursors to default", "-check", "-write center.Y", "-copy cursor 1", "-copy cursor 0", "-copy cursor 2", "move right", "move left", "shrink", "broaden", "skew up", "skew down", "-write plot scale", "zoom X", "change cen&win", "zoom to all data", "color--red", "color--green", "color--yellow", "read", "zoom out", "zoom in", "slide right", "slide left", "set range aspect ratio to 1"]
        n86 = call "cursor window action stack.vi"("stack action"=stack_action_--_control."push", "action list"=w224, "command stack"=w227) -> ("command stack out"=w226:T3[])  [unwired: 6 in, 2 out]
      }
      frame "set y to middle" {
        w231 = T3[] [enum."-read plot scale", enum."-set y to middle", enum."-write all Y"] items=["balance", "h. offset change", "cursor moves", "change center", "change window", "init", "check", "reset", "set y to middle", "idle", "-write all Y", "-write left.X", "-write center.X", "-write right.X", "-write all X", "-change center", "-change window", "-change skew", "-read cursor 2", "-read cursor 1", "-read cursor 0", "-read all cursors", "-reset", "-read plot scale", "-set y to middle", "-Q: center.Y is visible", "-Q: window is visible", "-parse center.Y", "-right left from center", "-left move", "-right move", "-set center.Y", "-empty", "-set cursors to default", "-check", "-write center.Y", "-copy cursor 1", "-copy cursor 0", "-copy cursor 2", "move right", "move left", "shrink", "broaden", "skew up", "skew down", "-write plot scale", "zoom X", "change cen&win", "zoom to all data", "color--red", "color--green", "color--yellow", "read", "zoom out", "zoom in", "slide right", "slide left", "set range aspect ratio to 1"]
        n87 = call "cursor window action stack.vi"("stack action"=stack_action_--_control."push", "action list"=w231, "command stack"=w234) -> ("command stack out"=w233:T3[])  [unwired: 6 in, 2 out]
      }
      frame "-left move" {
        n88 = Unbundle By Name(w247) -> ("center"=w240:dbl, "skew.left"=w243:dbl, "skew.right"=w242:dbl)
        n89 = Unbundle By Name(w245) -> ("left.X"=w241:dbl)
        n90 = call "Q -- check range -- i -- real.vi"("upper"=w240, "number"=w241) -> ("selector"=w239:T1)  [unwired: 7 in, 2 out]
        n91 = case shown="\"in range\", Default" w239 {
          tunnel: w241 -> [w252 w270]
          tunnel: w242 -> [w258 w269]
          tunnel: [w259 w268] -> w248
          tunnel: [w254 w263] -> w250
          tunnel: w243 -> [w260 w267]
          tunnel: [w256 w262] -> w249
          tunnel: w240 -> [w253 w266]
          tunnel: [enum16{"forw", "back"}."forw" ("wing order") enum16{"forw", "back"}."back" ("wing order")] -> w238
          frame "in range", Default {
            # "right wing"
            # "left wing"
            n92 = Subtract(x=w253, y=w252) -> (x-y=w257:dbl)
            n93 = Divide(x=w257, y=w260) -> (x/y=w259:dbl)
            n94 = Multiply(x=w259, y=w258) -> (x*y=w255:dbl)
            n95 = Subtract(x=w253, y=w257) -> (x-y=w256:dbl)
            n96 = Add(x=w255, y=w253) -> (x+y=w254:dbl)
          }
          frame "above" {
            # "right wing"
            # "left wing"
            n97 = Subtract(x=w270, y=w266) -> (x-y=w265:dbl)
            n98 = Divide(x=w265, y=w269) -> (x/y=w268:dbl)
            n99 = Multiply(x=w268, y=w267) -> (x*y=w264:dbl)
            n100 = Subtract(x=w266, y=w264) -> (x-y=w262:dbl)
            n101 = Add(x=w265, y=w266) -> (x+y=w263:dbl)
          }
        }
        n102 = Bundle By Name(cluster=w247, "left"=w249, "right"=w250, "window"=w248, "wing order"=w238) -> (w237:T2)
      }
      frame "-right move" {
        n103 = Unbundle By Name(w281) -> ("center"=w272:dbl, "skew.left"=w277:dbl, "skew.right"=w276:dbl)
        n104 = Unbundle By Name(w279) -> ("right.X"=w275:dbl)
        n105 = call "Q -- check range -- i -- real.vi"("lower"=w272, "number"=w275) -> ("selector"=w274:T1)  [unwired: 7 in, 2 out]
        n106 = case shown="\"below\"" w274 {
          tunnel: w275 -> [w294 w296]
          tunnel: w276 -> [w293 w302]
          tunnel: [w292 w303] -> w282
          tunnel: [w287 w298] -> w284
          tunnel: w277 -> [w291 w304]
          tunnel: [w286 w300] -> w283
          tunnel: w272 -> [w290 w297]
          tunnel: [enum16{"forw", "back"}."forw" ("wing order") enum16{"forw", "back"}."back" ("wing order")] -> w273
          frame "in range", Default {
            # "right wing"
            n107 = Subtract(x=w294, y=w290) -> (x-y=w289:dbl)
            n108 = Divide(x=w289, y=w293) -> (x/y=w292:dbl)
            n109 = Multiply(x=w292, y=w291) -> (x*y=w288:dbl)
            n110 = Subtract(x=w290, y=w288) -> (x-y=w286:dbl)
            n111 = Add(x=w289, y=w290) -> (x+y=w287:dbl)
          }
          frame "below" {
            # "right wing"
            # "left wing"
            n112 = Subtract(x=w297, y=w296) -> (x-y=w301:dbl)
            n113 = Divide(x=w301, y=w304) -> (x/y=w303:dbl)
            n114 = Multiply(x=w303, y=w302) -> (x*y=w299:dbl)
            n115 = Subtract(x=w297, y=w301) -> (x-y=w300:dbl)
            n116 = Add(x=w299, y=w297) -> (x+y=w298:dbl)
          }
        }
        n117 = Bundle By Name(cluster=w281, "left"=w283, "right"=w284, "window"=w282, "wing order"=w273) -> (w271:T2)
      }
      frame "-set center.Y" {
        # "zero"
        # "calculate center.Y   from"
        # "complementary to calculation of fraction from vert offset"
        n118 = Unbundle By Name(w322) -> ("scale.y.halfwidth"=w319:dbl, "scale.y.center"=w320:dbl, "scale.x.range"=w326:dbl, "scale.y.max"=w325:dbl, "scale.y.min"=w324:dbl)
        n119 = Unbundle By Name(w316) -> ("window"=w327:dbl, "fixed vertical offset"=w328:dbl, "kind"=w306:enum16{"symmetric", "skewed", "fancy"}, "default window frac"=w329:dbl, "skew"=w305:dbl)
        n120 = case shown="\"symmetric\", Default" w306 {
          tunnel: w329 -> [w341 _]
          tunnel: w327 -> [w340 _]
          tunnel: w326 -> [w339 _]
          tunnel: [w330 w342] -> w307
          tunnel: w305 -> [_ w342]
          frame "symmetric", Default {
            # "window fraction"
            # "-1..1"
            n121 = Multiply(x=w339, y=w341) -> (x*y=w335:dbl)
            n122 = Divide(x=w340, y=w335) -> (x/y=w334:dbl)
            n123 = call "Q -- check range -- i -- real.vi"("upper"=0.99 ("y"), "lower"=0.0 ("y"), "number"=w334) -> ("number in range"=w331:dbl)  [unwired: 6 in, 2 out]
            n124 = Multiply(x=2.0, y=w331) -> (x*y=w338:dbl)
            n125 = Subtract(x=w338, y=1.0) -> (x-y=w330:dbl)
          }
          frame "skewed" {
          }
        }
        n126 = Multiply(x=w328, y=1.0) -> (x*y=w310:dbl)
        n127 = Multiply(x=w310, y=w319) -> (x*y=w315:dbl)
        n128 = Add(x=w320, y=w315) -> (x+y=w308:dbl)
        n129 = Subtract(x=w308, y=w324) -> (x-y=w313:dbl)
        n130 = Subtract(x=w325, y=w308) -> (x-y=w314:dbl)
        n131 = Max & Min(x=w314, y=w313) -> (min(x,y)=w312:dbl)  [unwired: 1 out]
        n132 = Multiply(x=w312, y=w307) -> (x*y=w309:dbl)
        n133 = Add(x=w308, y=w309) -> (x+y=w323:dbl)
        n134 = Bundle By Name(cluster=w322, "center.Y"=w323) -> (w321:T4)
      }
      frame "cursor moves" {
        n135 = Unbundle By Name(w355) -> ("cursors"=w354:i32[], "kind"=w345:enum16{"symmetric", "skewed", "fancy"})
        n136 = case shown="\"fancy\"" w345 {
          tunnel: [w357 w361] -> w344
          tunnel: w343 -> [w357 w360]
          frame "symmetric", Default {
          }
          frame "fancy" {
            n137 = call "cursor window action stack.vi"("stack action"=stack_action_--_control."push", "cursor window action"=cursor_window_action."-write plot scale", "command stack"=w360) -> ("command stack out"=w361:T3[])  [unwired: 6 in, 2 out]
          }
        }
        n138 = Array Max & Min(array=w354) -> (max value=w352:i32, min value=w351:i32)  [unwired: 2 out]
        n139 = call "Q -- check range -- i -- integer.vi"("upper"=w352, "lower"=w351, "number"=w346) -> ("in range?"=w350:bool)  [unwired: 6 in, 2 out]
        n140 = Subtract(x=w346, y=w351) -> (x-y=w353:i32)
        n141 = case shown="True" w350 {
          tunnel: w344 -> [w363 w370]
          tunnel: [w363 w369] -> w356
          tunnel: w355 -> [w362 w368]
          tunnel: [w362 w367] -> w347
          tunnel: w354 -> [_ w366]
          tunnel: w353 -> [_ w365]
          frame False {
          }
          frame True {
            n142 = Index Array(array=w366, index=w365) -> (element=w364:i32)
            n143 = Bundle By Name(cluster=w368, "absolute"=w364, "relative"=w365) -> (w367:T2)
            n144 = case shown="0, 2, Default" w365 {
              selector: w365 -> [_ w380]
              tunnel: w370 -> [w374 w382]
              tunnel: [w373 w381] -> w369
              frame 1 {
                w371 = T3[] [enum."-read cursor 1", enum."-read plot scale", enum."-parse center.Y", enum."-copy cursor 1", enum."-change center", enum."-write right.X", enum."-write left.X"] items=["balance", "h. offset change", "cursor moves", "change center", "change window", "init", "check", "reset", "set y to middle", "idle", "-write all Y", "-write left.X", "-write center.X", "-write right.X", "-write all X", "-change center", "-change window", "-change skew", "-read cursor 2", "-read cursor 1", "-read cursor 0", "-read all cursors", "-reset", "-read plot scale", "-set y to middle", "-Q: center.Y is visible", "-Q: window is visible", "-parse center.Y", "-right left from center", "-left move", "-right move", "-set center.Y", "-empty", "-set cursors to default", "-check", "-write center.Y", "-copy cursor 1", "-copy cursor 0", "-copy cursor 2", "move right", "move left", "shrink", "broaden", "skew up", "skew down", "-write plot scale", "zoom X", "change cen&win", "zoom to all data", "color--red", "color--green", "color--yellow", "read", "zoom out", "zoom in", "slide right", "slide left", "set range aspect ratio to 1"]
                n145 = call "cursor window action stack.vi"("stack action"=stack_action_--_control."push", "action list"=w371, "command stack"=w374) -> ("command stack out"=w373:T3[])  [unwired: 6 in, 2 out]
              }
              frame 0, 2, Default {
                w379 = T3[] [enum."-set center.Y", enum."-write center.Y"] items=["balance", "h. offset change", "cursor moves", "change center", "change window", "init", "check", "reset", "set y to middle", "idle", "-write all Y", "-write left.X", "-write center.X", "-write right.X", "-write all X", "-change center", "-change window", "-change skew", "-read cursor 2", "-read cursor 1", "-read cursor 0", "-read all cursors", "-reset", "-read plot scale", "-set y to middle", "-Q: center.Y is visible", "-Q: window is visible", "-parse center.Y", "-right left from center", "-left move", "-right move", "-set center.Y", "-empty", "-set cursors to default", "-check", "-write center.Y", "-copy cursor 1", "-copy cursor 0", "-copy cursor 2", "move right", "move left", "shrink", "broaden", "skew up", "skew down", "-write plot scale", "zoom X", "change cen&win", "zoom to all data", "color--red", "color--green", "color--yellow", "read", "zoom out", "zoom in", "slide right", "slide left", "set range aspect ratio to 1"]
                w377 = T3[] [enum."-read plot scale"] items=["balance", "h. offset change", "cursor moves", "change center", "change window", "init", "check", "reset", "set y to middle", "idle", "-write all Y", "-write left.X", "-write center.X", "-write right.X", "-write all X", "-change center", "-change window", "-change skew", "-read cursor 2", "-read cursor 1", "-read cursor 0", "-read all cursors", "-reset", "-read plot scale", "-set y to middle", "-Q: center.Y is visible", "-Q: window is visible", "-parse center.Y", "-right left from center", "-left move", "-right move", "-set center.Y", "-empty", "-set cursors to default", "-check", "-write center.Y", "-copy cursor 1", "-copy cursor 0", "-copy cursor 2", "move right", "move left", "shrink", "broaden", "skew up", "skew down", "-write plot scale", "zoom X", "change cen&win", "zoom to all data", "color--red", "color--green", "color--yellow", "read", "zoom out", "zoom in", "slide right", "slide left", "set range aspect ratio to 1"]
                n146 = case shown="0, Default" w380 {
                  tunnel: [w383 w384] -> w378
                  frame 0, Default {
                    w383 = T3[] [enum."-read cursor 0", enum."-left move", enum."-write right.X"] items=["balance", "h. offset change", "cursor moves", "change center", "change window", "init", "check", "reset", "set y to middle", "idle", "-write all Y", "-write left.X", "-write center.X", "-write right.X", "-write all X", "-change center", "-change window", "-change skew", "-read cursor 2", "-read cursor 1", "-read cursor 0", "-read all cursors", "-reset", "-read plot scale", "-set y to middle", "-Q: center.Y is visible", "-Q: window is visible", "-parse center.Y", "-right left from center", "-left move", "-right move", "-set center.Y", "-empty", "-set cursors to default", "-check", "-write center.Y", "-copy cursor 1", "-copy cursor 0", "-copy cursor 2", "move right", "move left", "shrink", "broaden", "skew up", "skew down", "-write plot scale", "zoom X", "change cen&win", "zoom to all data", "color--red", "color--green", "color--yellow", "read", "zoom out", "zoom in", "slide right", "slide left", "set range aspect ratio to 1"]
                  }
                  frame 2 {
                    w384 = T3[] [enum."-read cursor 2", enum."-right move", enum."-write left.X"] items=["balance", "h. offset change", "cursor moves", "change center", "change window", "init", "check", "reset", "set y to middle", "idle", "-write all Y", "-write left.X", "-write center.X", "-write right.X", "-write all X", "-change center", "-change window", "-change skew", "-read cursor 2", "-read cursor 1", "-read cursor 0", "-read all cursors", "-reset", "-read plot scale", "-set y to middle", "-Q: center.Y is visible", "-Q: window is visible", "-parse center.Y", "-right left from center", "-left move", "-right move", "-set center.Y", "-empty", "-set cursors to default", "-check", "-write center.Y", "-copy cursor 1", "-copy cursor 0", "-copy cursor 2", "move right", "move left", "shrink", "broaden", "skew up", "skew down", "-write plot scale", "zoom X", "change cen&win", "zoom to all data", "color--red", "color--green", "color--yellow", "read", "zoom out", "zoom in", "slide right", "slide left", "set range aspect ratio to 1"]
                  }
                }
                n147 = Build Array (concatenate)(w377, w378, w379) -> (w375:T3[])
                n148 = call "cursor window action stack.vi"("stack action"=stack_action_--_control."push", "action list"=w375, "command stack"=w382) -> ("command stack out"=w381:T3[])  [unwired: 6 in, 2 out]
              }
            }
          }
        }
      }
      frame "idle" {
      }
      frame "-copy cursor 1" {
        n149 = Unbundle By Name(w394) -> ("center.X"=w393:dbl)
        n150 = Bundle By Name(cluster=w391, "center"=w393) -> (w390:T2)
      }
      frame "-set y to middle" {
        w395 = 0.5
        n151 = Unbundle By Name(w398) -> ("fixed vertical offset"=w404:dbl)
        n152 = Unbundle By Name(w403) -> ("scale.y.center"=w399:dbl, "scale.y.halfwidth"=w400:dbl)
        n153 = Multiply(x=w400, y=w404) -> (x*y=w405:dbl)
        n154 = Bundle By Name(cluster=w398, "skew"=0.0, "skew.left"=w395, "skew.right"=w395) -> (w397:T2)
        n155 = Add(x=w399, y=w405) -> (x+y=w401:dbl)
        n156 = Bundle By Name(cluster=w403, "right.Y"=w401, "center.Y"=w401, "left.Y"=w401) -> (w402:T4)
      }
      frame "-set cursors to default" {
        w411 = 0.5
        w410 = 0.1
        (unwired) 3
        n157 = Unbundle By Name(w421) -> ("scale.x.halfwidth"=w409:dbl, "scale.x.center"=w415:dbl)
        n158 = Multiply(x=w409, y=w410) -> (x*y=w408:dbl)
        n159 = Multiply(x=w408, y=2) -> (x*y=w414:dbl)
        n160 = Add(x=w415, y=w408) -> (x+y=w419:dbl)
        n161 = Subtract(x=w415, y=w408) -> (x-y=w420:dbl)
        n162 = Bundle By Name(cluster=w417, "vertical offset"=0.0, "default window frac"=w410, "left"=w420, "right"=w419, "center"=w415, "window"=w414, "skew"=0.0, "skew.left"=w411, "skew.right"=w411) -> (w413:T2)
      }
      frame "-read plot scale" {
        w435 = 2.0 ("y")
        w440 = 2.0 ("y")
        n163 = Unbundle By Name(w431) -> ("Plot ref"=w430:refnum<vi>)
        n164 = call "replace cursor - plot ref - V2.vi"("Plot ref in"=w430, "cursor action"=cursor_action."check") -> ("2Dwindow bounds out"=w429:T12)  [unwired: 14 in, 3 out]
        n165 = Unbundle By Name(w429) -> ("max y"=w428:dbl, "min y"=w427:dbl, "max x"=w426:dbl, "min x"=w425:dbl)
        n166 = Add(x=w426, y=w425) -> (x+y=w441:dbl)
        n167 = Subtract(x=w426, y=w425) -> (x-y=w439:dbl)
        n168 = Divide(x=w441, y=w440) -> (x/y=w438:dbl)
        n169 = Divide(x=w439, y=w440) -> (x/y=w437:dbl)
        n170 = Subtract(x=w428, y=w427) -> (x-y=w432:dbl)
        n171 = Add(x=w428, y=w427) -> (x+y=w436:dbl)
        n172 = Divide(x=w436, y=w435) -> (x/y=w434:dbl)
        n173 = Divide(x=w432, y=w435) -> (x/y=w433:dbl)
        n174 = Bundle By Name(cluster=w444, "scale.y.max"=w428, "scale.y.min"=w427, "scale.x.max"=w426, "scale.x.min"=w425, "scale.x.range"=w439, "scale.x.halfwidth"=w437, "scale.x.center"=w438, "scale.y.range"=w432, "scale.y.halfwidth"=w433, "scale.y.center"=w434) -> (w443:T4)
      }
      frame "-write plot scale" {
        n175 = Unbundle By Name(w457) -> ("Plot ref"=w450:refnum<vi>, "window"=w454:dbl, "center"=w453:dbl, "default window frac"=w452:dbl)
        n176 = call "Q -- range multiplier -- real -- V2.vi"("factor"=w452, "rage multiplier action"=range_multiplier_action."zoom", "center"=w453, "window"=w454) -> ("center OUT"=w448:dbl, "window OUT"=w447:dbl)  [unwired: 4 in, 2 out]
        n177 = Bundle By Name(cluster=T10 {"window y"=0.0021014740628288917, "center x"=44850.89441339177, "center y"=2.5658109925320947, "window x"=17480.201988350764} ("window IN"), "window x"=w447, "center x"=w448) -> (w446:T10)
        n178 = call "replace cursor - plot ref - V2.vi"("Plot ref in"=w450, "window IN"=w446, "cursor action"=cursor_action."zoom to X win") -> ()  [unwired: 13 in, 4 out]
      }
      frame "zoom X" {
        n179 = Unbundle By Name(w472) -> ("Plot ref"=w464:refnum<vi>, "window"=w463:dbl, "center"=w462:dbl, "default window frac"=w461:dbl)
        n180 = Reciprocal(x=w461) -> (1/x=w460:dbl)
        n181 = call "Q -- range multiplier -- real -- V2.vi"("factor"=w460, "rage multiplier action"=range_multiplier_action."zoom", "center"=w462, "window"=w463) -> ("center OUT"=w467:dbl, "window OUT"=w466:dbl)  [unwired: 4 in, 2 out]
        n182 = Bundle By Name(cluster=T10 {"window y"=0.0021014740628288917, "center x"=44850.89441339177, "center y"=2.5658109925320947, "window x"=17480.201988350764} ("window IN"), "window x"=w466, "center x"=w467) -> (w465:T10)
        n183 = call "replace cursor - plot ref - V2.vi"("Plot ref in"=w464, "window IN"=w465, "cursor action"=cursor_action."zoom to X win") -> ()  [unwired: 13 in, 4 out]
      }
      frame "zoom out" {
        (unwired) range_multiplier_action."zoom" ("rage multiplier action")
        n184 = Unbundle By Name(w478) -> ("Plot ref"=w475:refnum<vi>)
        n185 = call "replace cursor - plot ref - V2.vi"("Plot ref in"=w475, "cursor action"=cursor_action."zoom out X") -> ()  [unwired: 14 in, 4 out]
      }
      frame "set range aspect ratio to 1" {
        n186 = Unbundle By Name(w484) -> ("Plot ref"=w482:refnum<vi>)
        n187 = call "replace cursor - plot ref - V2.vi"("Plot ref in"=w482, "cursor action"=cursor_action."zoom to aspect ratio 1") -> ()  [unwired: 14 in, 4 out]
      }
      frame "zoom in" {
        n188 = Unbundle By Name(w490) -> ("Plot ref"=w488:refnum<vi>)
        n189 = call "replace cursor - plot ref - V2.vi"("Plot ref in"=w488, "cursor action"=cursor_action."zoom in X") -> ()  [unwired: 14 in, 4 out]
      }
      frame "slide right" {
        n190 = Unbundle By Name(w496) -> ("Plot ref"=w494:refnum<vi>)
        n191 = call "replace cursor - plot ref - V2.vi"("Plot ref in"=w494, "cursor action"=cursor_action."move range right 20%") -> ()  [unwired: 14 in, 4 out]
      }
      frame "slide left" {
        n192 = Unbundle By Name(w502) -> ("Plot ref"=w500:refnum<vi>)
        n193 = call "replace cursor - plot ref - V2.vi"("Plot ref in"=w500, "cursor action"=cursor_action."move range left 20%") -> ()  [unwired: 14 in, 4 out]
      }
      frame "-Q: center.Y is visible" {
        # "check if y is within y-scale bounds"
        n194 = Unbundle By Name(w511) -> ("center.Y"=w514:dbl, "scale.y.max"=w513:dbl, "scale.y.min"=w512:dbl, "scale.y.center"=w505:dbl)
        n195 = call "Q -- check range -- i -- real.vi"("upper"=w513, "lower"=w512, "number"=w514) -> ("in range?"=w506:bool)  [unwired: 6 in, 2 out]
        n196 = case shown="False" w506 {
          tunnel: w511 -> [w522 w524]
          tunnel: [w521 w524] -> w510
          tunnel: w508 -> [w519 w523]
          tunnel: [w517 w523] -> w507
          tunnel: w505 -> [w516 _]
          frame False {
            w520 = T3[] [enum."-parse center.Y", enum."-write center.Y"] items=["balance", "h. offset change", "cursor moves", "change center", "change window", "init", "check", "reset", "set y to middle", "idle", "-write all Y", "-write left.X", "-write center.X", "-write right.X", "-write all X", "-change center", "-change window", "-change skew", "-read cursor 2", "-read cursor 1", "-read cursor 0", "-read all cursors", "-reset", "-read plot scale", "-set y to middle", "-Q: center.Y is visible", "-Q: window is visible", "-parse center.Y", "-right left from center", "-left move", "-right move", "-set center.Y", "-empty", "-set cursors to default", "-check", "-write center.Y", "-copy cursor 1", "-copy cursor 0", "-copy cursor 2", "move right", "move left", "shrink", "broaden", "skew up", "skew down", "-write plot scale", "zoom X", "change cen&win", "zoom to all data", "color--red", "color--green", "color--yellow", "read", "zoom out", "zoom in", "slide right", "slide left", "set range aspect ratio to 1"]
            n197 = Bundle By Name(cluster=w522, "center.Y"=w516) -> (w521:T4)
            n198 = call "cursor window action stack.vi"("stack action"=stack_action_--_control."push", "action list"=w520, "command stack"=w519) -> ("command stack out"=w517:T3[])  [unwired: 6 in, 2 out]
          }
          frame True {
          }
        }
      }
      frame "move left" {
        (unwired) 0.2
        w537 = T3[] [enum."-change center", enum."-write all X"] items=["balance", "h. offset change", "cursor moves", "change center", "change window", "init", "check", "reset", "set y to middle", "idle", "-write all Y", "-write left.X", "-write center.X", "-write right.X", "-write all X", "-change center", "-change window", "-change skew", "-read cursor 2", "-read cursor 1", "-read cursor 0", "-read all cursors", "-reset", "-read plot scale", "-set y to middle", "-Q: center.Y is visible", "-Q: window is visible", "-parse center.Y", "-right left from center", "-left move", "-right move", "-set center.Y", "-empty", "-set cursors to default", "-check", "-write center.Y", "-copy cursor 1", "-copy cursor 0", "-copy cursor 2", "move right", "move left", "shrink", "broaden", "skew up", "skew down", "-write plot scale", "zoom X", "change cen&win", "zoom to all data", "color--red", "color--green", "color--yellow", "read", "zoom out", "zoom in", "slide right", "slide left", "set range aspect ratio to 1"]
        n199 = Unbundle By Name(w533) -> ("center"=w527:dbl, "window"=w526:dbl, "default window frac"=w525:dbl)  [unwired: 1 out]
        n200 = Multiply(x=w526, y=w525) -> (x*y=w528:dbl)
        n201 = Subtract(x=w527, y=w528) -> (x-y=w531:dbl)
        n202 = Bundle By Name(cluster=w533, "center"=w531) -> (w532:T2)
        n203 = call "cursor window action stack.vi"("stack action"=stack_action_--_control."push", "action list"=w537, "command stack"=w535) -> ("command stack out"=w534:T3[])  [unwired: 6 in, 2 out]
      }
      frame "move right" {
        (unwired) 0.2
        w550 = T3[] [enum."-change center", enum."-write all X"] items=["balance", "h. offset change", "cursor moves", "change center", "change window", "init", "check", "reset", "set y to middle", "idle", "-write all Y", "-write left.X", "-write center.X", "-write right.X", "-write all X", "-change center", "-change window", "-change skew", "-read cursor 2", "-read cursor 1", "-read cursor 0", "-read all cursors", "-reset", "-read plot scale", "-set y to middle", "-Q: center.Y is visible", "-Q: window is visible", "-parse center.Y", "-right left from center", "-left move", "-right move", "-set center.Y", "-empty", "-set cursors to default", "-check", "-write center.Y", "-copy cursor 1", "-copy cursor 0", "-copy cursor 2", "move right", "move left", "shrink", "broaden", "skew up", "skew down", "-write plot scale", "zoom X", "change cen&win", "zoom to all data", "color--red", "color--green", "color--yellow", "read", "zoom out", "zoom in", "slide right", "slide left", "set range aspect ratio to 1"]
        n204 = Unbundle By Name(w539) -> ("center"=w542:dbl, "window"=w541:dbl, "default window frac"=w540:dbl)  [unwired: 1 out]
        n205 = Multiply(x=w541, y=w540) -> (x*y=w543:dbl)
        n206 = Add(x=w542, y=w543) -> (x+y=w544:dbl)
        n207 = Bundle By Name(cluster=w539, "center"=w544) -> (w538:T2)
        n208 = call "cursor window action stack.vi"("stack action"=stack_action_--_control."push", "action list"=w550, "command stack"=w548) -> ("command stack out"=w547:T3[])  [unwired: 6 in, 2 out]
      }
      frame "shrink" {
        (unwired) 0.3
        w563 = T3[] [enum."-change window", enum."-write all X", enum."-read plot scale", enum."-set center.Y", enum."-write center.Y"] items=["balance", "h. offset change", "cursor moves", "change center", "change window", "init", "check", "reset", "set y to middle", "idle", "-write all Y", "-write left.X", "-write center.X", "-write right.X", "-write all X", "-change center", "-change window", "-change skew", "-read cursor 2", "-read cursor 1", "-read cursor 0", "-read all cursors", "-reset", "-read plot scale", "-set y to middle", "-Q: center.Y is visible", "-Q: window is visible", "-parse center.Y", "-right left from center", "-left move", "-right move", "-set center.Y", "-empty", "-set cursors to default", "-check", "-write center.Y", "-copy cursor 1", "-copy cursor 0", "-copy cursor 2", "move right", "move left", "shrink", "broaden", "skew up", "skew down", "-write plot scale", "zoom X", "change cen&win", "zoom to all data", "color--red", "color--green", "color--yellow", "read", "zoom out", "zoom in", "slide right", "slide left", "set range aspect ratio to 1"]
        n209 = Unbundle By Name(w559) -> ("window"=w554:dbl, "window"=w553:dbl, "default window frac"=w551:dbl)
        n210 = Multiply(x=w553, y=w551) -> (x*y=w552:dbl)
        n211 = Subtract(x=w554, y=w552) -> (x-y=w557:dbl)
        n212 = Bundle By Name(cluster=w559, "window"=w557) -> (w558:T2)
        n213 = call "cursor window action stack.vi"("stack action"=stack_action_--_control."push", "action list"=w563, "command stack"=w561) -> ("command stack out"=w560:T3[])  [unwired: 6 in, 2 out]
      }
      frame "broaden" {
        (unwired) 0.3
        w571 = T3[] [enum."-change window", enum."-write all X", enum."-read plot scale", enum."-set center.Y", enum."-write center.Y"] items=["balance", "h. offset change", "cursor moves", "change center", "change window", "init", "check", "reset", "set y to middle", "idle", "-write all Y", "-write left.X", "-write center.X", "-write right.X", "-write all X", "-change center", "-change window", "-change skew", "-read cursor 2", "-read cursor 1", "-read cursor 0", "-read all cursors", "-reset", "-read plot scale", "-set y to middle", "-Q: center.Y is visible", "-Q: window is visible", "-parse center.Y", "-right left from center", "-left move", "-right move", "-set center.Y", "-empty", "-set cursors to default", "-check", "-write center.Y", "-copy cursor 1", "-copy cursor 0", "-copy cursor 2", "move right", "move left", "shrink", "broaden", "skew up", "skew down", "-write plot scale", "zoom X", "change cen&win", "zoom to all data", "color--red", "color--green", "color--yellow", "read", "zoom out", "zoom in", "slide right", "slide left", "set range aspect ratio to 1"]
        n214 = Unbundle By Name(w565) -> ("window"=w569:dbl, "window"=w568:dbl, "default window frac"=w566:dbl)
        n215 = Multiply(x=w568, y=w566) -> (x*y=w567:dbl)
        n216 = Add(x=w569, y=w567) -> (x+y=w570:dbl)
        n217 = Bundle By Name(cluster=w565, "window"=w570) -> (w564:T2)
        n218 = call "cursor window action stack.vi"("stack action"=stack_action_--_control."push", "action list"=w571, "command stack"=w575) -> ("command stack out"=w574:T3[])  [unwired: 6 in, 2 out]
      }
      frame "skew up" {
        n219 = Unbundle By Name(w578) -> ("kind"=w577:enum16{"symmetric", "skewed", "fancy"})
        n220 = case shown="\"skewed\"" w577 {
          tunnel: w583 -> [w585 w595]
          tunnel: [w585 w594] -> w582
          tunnel: [w584 w593] -> w581
          tunnel: w578 -> [w584 w591]
          frame "symmetric", Default {
          }
          frame "skewed" {
            w597 = T3[] [enum."-change skew", enum."-read plot scale", enum."-set center.Y", enum."-write right.X", enum."-write left.X", enum."-write center.Y"] items=["balance", "h. offset change", "cursor moves", "change center", "change window", "init", "check", "reset", "set y to middle", "idle", "-write all Y", "-write left.X", "-write center.X", "-write right.X", "-write all X", "-change center", "-change window", "-change skew", "-read cursor 2", "-read cursor 1", "-read cursor 0", "-read all cursors", "-reset", "-read plot scale", "-set y to middle", "-Q: center.Y is visible", "-Q: window is visible", "-parse center.Y", "-right left from center", "-left move", "-right move", "-set center.Y", "-empty", "-set cursors to default", "-check", "-write center.Y", "-copy cursor 1", "-copy cursor 0", "-copy cursor 2", "move right", "move left", "shrink", "broaden", "skew up", "skew down", "-write plot scale", "zoom X", "change cen&win", "zoom to all data", "color--red", "color--green", "color--yellow", "read", "zoom out", "zoom in", "slide right", "slide left", "set range aspect ratio to 1"]
            n221 = Unbundle By Name(w591) -> ("skew"=w592:dbl)
            n222 = Add(x=0.1, y=w592) -> (x+y=w589:dbl)
            n223 = call "Q -- check range -- i -- real.vi"("upper"=1, "lower"=-1, "number"=w589) -> ("number in range"=w586:dbl)  [unwired: 6 in, 2 out]
            n224 = Bundle By Name(cluster=w591, "skew"=w586) -> (w593:T2)
            n225 = call "cursor window action stack.vi"("stack action"=stack_action_--_control."push", "action list"=w597, "command stack"=w595) -> ("command stack out"=w594:T3[])  [unwired: 6 in, 2 out]
          }
        }
      }
      frame "skew down" {
        n226 = Unbundle By Name(w599) -> ("kind"=w598:enum16{"symmetric", "skewed", "fancy"})
        n227 = case shown="\"skewed\"" w598 {
          tunnel: w604 -> [w606 w617]
          tunnel: [w606 w616] -> w603
          tunnel: [w605 w615] -> w602
          tunnel: w599 -> [w605 w614]
          frame "symmetric", Default {
          }
          frame "skewed" {
            w609 = T3[] [enum."-change skew", enum."-read plot scale", enum."-set center.Y", enum."-write right.X", enum."-write left.X", enum."-write center.Y"] items=["balance", "h. offset change", "cursor moves", "change center", "change window", "init", "check", "reset", "set y to middle", "idle", "-write all Y", "-write left.X", "-write center.X", "-write right.X", "-write all X", "-change center", "-change window", "-change skew", "-read cursor 2", "-read cursor 1", "-read cursor 0", "-read all cursors", "-reset", "-read plot scale", "-set y to middle", "-Q: center.Y is visible", "-Q: window is visible", "-parse center.Y", "-right left from center", "-left move", "-right move", "-set center.Y", "-empty", "-set cursors to default", "-check", "-write center.Y", "-copy cursor 1", "-copy cursor 0", "-copy cursor 2", "move right", "move left", "shrink", "broaden", "skew up", "skew down", "-write plot scale", "zoom X", "change cen&win", "zoom to all data", "color--red", "color--green", "color--yellow", "read", "zoom out", "zoom in", "slide right", "slide left", "set range aspect ratio to 1"]
            n228 = Unbundle By Name(w614) -> ("skew"=w608:dbl)
            n229 = Subtract(x=w608, y=0.1) -> (x-y=w613:dbl)
            n230 = call "Q -- check range -- i -- real.vi"("upper"=1, "lower"=-1, "number"=w613) -> ("number in range"=w610:dbl)  [unwired: 6 in, 2 out]
            n231 = Bundle By Name(cluster=w614, "skew"=w610) -> (w615:T2)
            n232 = call "cursor window action stack.vi"("stack action"=stack_action_--_control."push", "action list"=w609, "command stack"=w617) -> ("command stack out"=w616:T3[])  [unwired: 6 in, 2 out]
          }
        }
      }
      frame "-parse center.Y" {
        w631 = 1.0  # y
        w633 = 2.0  # y
        # "left factor"
        # "right factor"
        # "0 .. 1"
        # "-1 .. 1"
        # "-1..1"
        # "\"zero\""
        # "calculate horizontal offset and/or window \nfrom vertical position of center cursor"
        n233 = Unbundle By Name(w642) -> ("center.Y"=w627:dbl, "scale.y.max"=w625:dbl, "scale.y.min"=w626:dbl, "scale.y.center"=w623:dbl, "scale.y.halfwidth"=w635:dbl)
        n234 = Unbundle By Name(w638) -> ("fixed vertical offset"=w655:dbl)
        n235 = Multiply(x=w635, y=w655) -> (x*y=w653:dbl)
        n236 = call "Q -- check range -- i -- real.vi"("upper"=w625, "lower"=w626, "default"=w623, "number"=w627) -> ("number in range"=w624:dbl)  [unwired: 5 in, 2 out]
        n237 = Add(x=w653, y=w623) -> (x+y=w650:dbl)
        n238 = Unbundle By Name(w638) -> ("default window frac"=w643:dbl, "kind"=w644:enum16{"symmetric", "skewed", "fancy"}, "skew"=w640:dbl, "window"=w639:dbl)
        n239 = Unbundle By Name(w642) -> ("scale.x.range"=w641:dbl)
        n240 = Subtract(x=w650, y=w626) -> (x-y=w651:dbl)
        n241 = Subtract(x=w625, y=w650) -> (x-y=w652:dbl)
        n242 = Max & Min(x=w652, y=w651) -> (min(x,y)=w648:dbl)  [unwired: 1 out]
        n243 = Subtract(x=w624, y=w650) -> (x-y=w649:dbl)
        n244 = Divide(x=w649, y=w648) -> (x/y=w647:dbl)
        n245 = Multiply(x=w647, y=0.99) -> (x*y=w622:dbl)
        n246 = call "Q -- check range -- i -- real.vi"("upper"=1, "lower"=-1, "number"=w622) -> ("number in range"=w619:dbl)  [unwired: 6 in, 2 out]
        n247 = Bundle By Name(cluster=w642, "center.Y"=w624) -> (w645:T4)
        n248 = case shown="\"symmetric\", Default" w644 {
          tunnel: [w656 w667] -> w630
          tunnel: w619 -> [w665 w667]
          tunnel: w643 -> [w664 _]
          tunnel: w641 -> [w663 _]
          tunnel: [w657 w666] -> w637
          tunnel: w640 -> [w656 _]
          tunnel: w639 -> [_ w666]
          frame "symmetric", Default {
            # "0 .. 1"
            # "-1 .. 1"
            n249 = Add(x=w665, y=1.0) -> (x+y=w661:dbl)
            n250 = Divide(x=w661, y=2.0) -> (x/y=w659:dbl)
            n251 = Multiply(x=w664, y=w659) -> (x*y=w658:dbl)
            n252 = Multiply(x=w658, y=w663) -> (x*y=w657:dbl)
          }
          frame "skewed" {
          }
        }
        n253 = Add(x=w630, y=w631) -> (x+y=w632:dbl)
        n254 = Divide(x=w632, y=w633) -> (x/y=w628:dbl)
        n255 = Subtract(x=w631, y=w628) -> (x-y=w629:dbl)
        n256 = Bundle By Name(cluster=w638, "skew"=w630, "window"=w637, "skew.left"=w629, "skew.right"=w628) -> (w634:T2)
      }
      frame "-Q: window is visible" {
        n257 = Unbundle By Name(w678) -> ("scale.x.min"=w670:dbl, "scale.x.max"=w669:dbl, "scale.x.center"=w673:dbl, "scale.x.range"=w668:dbl)  [unwired: 1 out]
        n258 = Unbundle By Name(w672) -> ("center"=w677:dbl)
        n259 = call "Q -- check range -- i -- real.vi"("upper"=w669, "lower"=w670, "number"=w677) -> ("selector"=w676:T1)  [unwired: 6 in, 2 out]
        "selector" <- w676
        n260 = case shown="\"in range\"" w676 {
          tunnel: w675 -> [w685 w710]
          tunnel: [w684 w708] -> w674
          tunnel: w672 -> [w683 w707]
          tunnel: w673 -> [_ w706]
          tunnel: [w681 w705] -> w671
          tunnel: w670 -> [w691 _]
          tunnel: w669 -> [w690 _]
          tunnel: w668 -> [w682 _]
          frame "in range" {
            n261 = Unbundle By Name(w683) -> ("left"=w693:dbl, "right"=w692:dbl)
            n262 = call "Q -- check range -- i -- real.vi"("upper"=w690, "lower"=w691, "number"=w693) -> ("in range?"=w689:bool)  [unwired: 6 in, 2 out]
            n263 = call "Q -- check range -- i -- real.vi"("upper"=w690, "lower"=w691, "number"=w692) -> ("in range?"=w688:bool)  [unwired: 6 in, 2 out]
            n264 = Not(x=w689) -> (.not. x?=w687:bool)
            n265 = Not(x=w688) -> (.not. x?=w686:bool)
            n266 = And(x=w687, y=w686) -> (x .and. y?=w680:bool)
            n267 = case shown="True" w680 {
              tunnel: w685 -> [w695 w702]
              tunnel: [w695 w701] -> w684
              tunnel: w683 -> [w694 w700]
              tunnel: w682 -> [_ w698]
              tunnel: [w694 w696] -> w681
              frame False {
              }
              frame True {
                w704 = T3[] [enum."-change window", enum."-write left.X", enum."-write right.X"] items=["balance", "h. offset change", "cursor moves", "change center", "change window", "init", "check", "reset", "set y to middle", "idle", "-write all Y", "-write left.X", "-write center.X", "-write right.X", "-write all X", "-change center", "-change window", "-change skew", "-read cursor 2", "-read cursor 1", "-read cursor 0", "-read all cursors", "-reset", "-read plot scale", "-set y to middle", "-Q: center.Y is visible", "-Q: window is visible", "-parse center.Y", "-right left from center", "-left move", "-right move", "-set center.Y", "-empty", "-set cursors to default", "-check", "-write center.Y", "-copy cursor 1", "-copy cursor 0", "-copy cursor 2", "move right", "move left", "shrink", "broaden", "skew up", "skew down", "-write plot scale", "zoom X", "change cen&win", "zoom to all data", "color--red", "color--green", "color--yellow", "read", "zoom out", "zoom in", "slide right", "slide left", "set range aspect ratio to 1"]
                n268 = Unbundle By Name(w700) -> ("default window frac"=w699:dbl)
                n269 = Multiply(x=w699, y=w698) -> (x*y=w697:dbl)
                n270 = Bundle By Name(cluster=w700, "window"=w697) -> (w696:T2)
                n271 = call "cursor window action stack.vi"("stack action"=stack_action_--_control."push", "action list"=w704, "command stack"=w702) -> ("command stack out"=w701:T3[])  [unwired: 6 in, 2 out]
              }
            }
          }
          frame "not a number", "above", "below", Default {
            w711 = T3[] [enum."-change center", enum."-write all X", enum."-Q: window is visible"] items=["balance", "h. offset change", "cursor moves", "change center", "change window", "init", "check", "reset", "set y to middle", "idle", "-write all Y", "-write left.X", "-write center.X", "-write right.X", "-write all X", "-change center", "-change window", "-change skew", "-read cursor 2", "-read cursor 1", "-read cursor 0", "-read all cursors", "-reset", "-read plot scale", "-set y to middle", "-Q: center.Y is visible", "-Q: window is visible", "-parse center.Y", "-right left from center", "-left move", "-right move", "-set center.Y", "-empty", "-set cursors to default", "-check", "-write center.Y", "-copy cursor 1", "-copy cursor 0", "-copy cursor 2", "move right", "move left", "shrink", "broaden", "skew up", "skew down", "-write plot scale", "zoom X", "change cen&win", "zoom to all data", "color--red", "color--green", "color--yellow", "read", "zoom out", "zoom in", "slide right", "slide left", "set range aspect ratio to 1"]
            n272 = Bundle By Name(cluster=w707, "center"=w706) -> (w705:T2)
            n273 = call "cursor window action stack.vi"("stack action"=stack_action_--_control."push", "action list"=w711, "command stack"=w710) -> ("command stack out"=w708:T3[])  [unwired: 6 in, 2 out]
          }
        }
      }
      frame "-write all X" {
        w728 = cursor_action."write"  # action
        n274 = Unbundle By Name(w712) -> ("Plot ref"=w713:refnum<vi>, "cursors"=w726:i32[], "left"=w720:dbl, "center"=w719:dbl, "right"=w718:dbl)
        n275 = Index Array(array=w726, index #1=0 ("cursor index"), index #2=1 ("cursor index"), index #3=2 ("cursor index")) -> (element #1=w727:i32, element #2=w723:i32, element #3=w721:i32)
        n276 = call "replace cursor - plot ref - V2.vi"("Plot ref in"=w713, "new X"=w720, "cursor index"=w727, "cursor action"=w728) -> ("Plot ref out"=w717:refnum<vi>)  [unwired: 12 in, 3 out]
        n277 = call "replace cursor - plot ref - V2.vi"("Plot ref in"=w717, "new X"=w719, "cursor index"=w723, "cursor action"=w728) -> ("Plot ref out"=w716:refnum<vi>)  [unwired: 12 in, 3 out]
        n278 = call "replace cursor - plot ref - V2.vi"("Plot ref in"=w716, "new X"=w718, "cursor index"=w721, "cursor action"=w728) -> ()  [unwired: 12 in, 4 out]
      }
      frame "color--red" {
        w730 = cursor_sate."colored" ("cursor state")
        w731 = u32 16728794 ("Color Box")
        w732 = cursor_action."write"  # action
        n279 = Unbundle By Name(w733) -> ("Plot ref"=w734:refnum<vi>, "cursors"=w747:i32[], "left"=w741:dbl, "center"=w740:dbl, "right"=w739:dbl)
        n280 = Index Array(array=w747, index #1=0 ("cursor index"), index #2=1 ("cursor index"), index #3=2 ("cursor index")) -> (element #1=w748:i32, element #2=w744:i32, element #3=w742:i32)
        n281 = call "replace cursor - plot ref - V2.vi"("Plot ref in"=w734, "new X"=w741, "cursor index"=w748, "cursor action"=w732, "Color Box"=w731, "cursor state"=w730) -> ("Plot ref out"=w738:refnum<vi>)  [unwired: 10 in, 3 out]
        n282 = call "replace cursor - plot ref - V2.vi"("Plot ref in"=w738, "new X"=w740, "cursor index"=w744, "cursor action"=w732, "Color Box"=w731, "cursor state"=w730) -> ("Plot ref out"=w737:refnum<vi>)  [unwired: 10 in, 3 out]
        n283 = call "replace cursor - plot ref - V2.vi"("Plot ref in"=w737, "new X"=w739, "cursor index"=w742, "cursor action"=w732, "Color Box"=w731, "cursor state"=w730) -> ()  [unwired: 10 in, 4 out]
      }
      frame "color--green" {
        w750 = cursor_sate."colored" ("cursor state")
        w751 = u32 4250624 ("Color Box")
        w752 = cursor_action."write"  # action
        n284 = Unbundle By Name(w753) -> ("Plot ref"=w754:refnum<vi>, "cursors"=w767:i32[], "left"=w761:dbl, "center"=w760:dbl, "right"=w759:dbl)
        n285 = Index Array(array=w767, index #1=0 ("cursor index"), index #2=1 ("cursor index"), index #3=2 ("cursor index")) -> (element #1=w768:i32, element #2=w764:i32, element #3=w762:i32)
        n286 = call "replace cursor - plot ref - V2.vi"("Plot ref in"=w754, "new X"=w761, "cursor index"=w768, "cursor action"=w752, "Color Box"=w751, "cursor state"=w750) -> ("Plot ref out"=w758:refnum<vi>)  [unwired: 10 in, 3 out]
        n287 = call "replace cursor - plot ref - V2.vi"("Plot ref in"=w758, "new X"=w760, "cursor index"=w764, "cursor action"=w752, "Color Box"=w751, "cursor state"=w750) -> ("Plot ref out"=w757:refnum<vi>)  [unwired: 10 in, 3 out]
        n288 = call "replace cursor - plot ref - V2.vi"("Plot ref in"=w757, "new X"=w759, "cursor index"=w762, "cursor action"=w752, "Color Box"=w751, "cursor state"=w750) -> ()  [unwired: 10 in, 4 out]
      }
      frame "color--yellow" {
        w770 = cursor_sate."colored" ("cursor state")
        w771 = u32 16773632 ("Color Box")
        w772 = cursor_action."write"  # action
        n289 = Unbundle By Name(w773) -> ("Plot ref"=w774:refnum<vi>, "cursors"=w787:i32[], "left"=w781:dbl, "center"=w780:dbl, "right"=w779:dbl)
        n290 = Index Array(array=w787, index #1=0 ("cursor index"), index #2=1 ("cursor index"), index #3=2 ("cursor index")) -> (element #1=w788:i32, element #2=w784:i32, element #3=w782:i32)
        n291 = call "replace cursor - plot ref - V2.vi"("Plot ref in"=w774, "new X"=w781, "cursor index"=w788, "cursor action"=w772, "Color Box"=w771, "cursor state"=w770) -> ("Plot ref out"=w778:refnum<vi>)  [unwired: 10 in, 3 out]
        n292 = call "replace cursor - plot ref - V2.vi"("Plot ref in"=w778, "new X"=w780, "cursor index"=w784, "cursor action"=w772, "Color Box"=w771, "cursor state"=w770) -> ("Plot ref out"=w777:refnum<vi>)  [unwired: 10 in, 3 out]
        n293 = call "replace cursor - plot ref - V2.vi"("Plot ref in"=w777, "new X"=w779, "cursor index"=w782, "cursor action"=w772, "Color Box"=w771, "cursor state"=w770) -> ()  [unwired: 10 in, 4 out]
      }
      frame "-write all Y" {
        w806 = cursor_action."write"  # action
        n294 = Unbundle By Name(w794) -> ("Plot ref"=w795:refnum<vi>, "cursors"=w804:i32[])
        n295 = Unbundle By Name(w793) -> ("left.Y"=w792:dbl, "center.Y"=w791:dbl, "right.Y"=w790:dbl)
        n296 = Index Array(array=w804, index #1=0 ("cursor index"), index #2=1 ("cursor index"), index #3=2 ("cursor index")) -> (element #1=w805:i32, element #2=w801:i32, element #3=w799:i32)
        n297 = call "replace cursor - plot ref - V2.vi"("Plot ref in"=w795, "new  Y"=w792, "cursor index"=w805, "cursor action"=w806) -> ("Plot ref out"=w798:refnum<vi>)  [unwired: 12 in, 3 out]
        n298 = call "replace cursor - plot ref - V2.vi"("Plot ref in"=w798, "new  Y"=w791, "cursor index"=w801, "cursor action"=w806) -> ("Plot ref out"=w797:refnum<vi>)  [unwired: 12 in, 3 out]
        n299 = call "replace cursor - plot ref - V2.vi"("Plot ref in"=w797, "new  Y"=w790, "cursor index"=w799, "cursor action"=w806) -> ()  [unwired: 12 in, 4 out]
      }
      frame "-write left.X" {
        w821 = cursor_action."write"  # action
        n300 = Unbundle By Name(w808) -> ("Plot ref"=w813:refnum<vi>, "cursors"=w819:i32[], "left"=w809:dbl, "right"=w810:dbl, "wing order"=w812:enum16{"forw", "back"})
        n301 = Index Array(array=w819, index #1=0 ("cursor index"), index #2=1 ("cursor index"), index #3=2 ("cursor index")) -> (element #1=w820:i32)  [unwired: 2 out]
        n302 = case shown="\"back\"" w812 {
          tunnel: [w823 w824] -> w811
          tunnel: w810 -> [_ w824]
          tunnel: w809 -> [w823 _]
          frame "forw", Default {
          }
          frame "back" {
          }
        }
        n303 = call "replace cursor - plot ref - V2.vi"("Plot ref in"=w813, "new X"=w811, "cursor index"=w820, "cursor action"=w821) -> ()  [unwired: 12 in, 4 out]
      }
      frame "-write right.X" {
        w838 = cursor_action."write"  # action
        n304 = Unbundle By Name(w825) -> ("Plot ref"=w831:refnum<vi>, "cursors"=w837:i32[], "left"=w827:dbl, "right"=w828:dbl, "wing order"=w830:enum16{"forw", "back"})
        n305 = Index Array(array=w837, index #1=0 ("cursor index"), index #2=1 ("cursor index"), index #3=2 ("cursor index")) -> (element #3=w826:i32)  [unwired: 2 out]
        n306 = case shown="\"back\"" w830 {
          tunnel: [w840 w841] -> w829
          tunnel: w828 -> [w840 _]
          tunnel: w827 -> [_ w841]
          frame "forw", Default {
          }
          frame "back" {
          }
        }
        n307 = call "replace cursor - plot ref - V2.vi"("Plot ref in"=w831, "new X"=w829, "cursor index"=w826, "cursor action"=w838) -> ()  [unwired: 12 in, 4 out]
      }
      frame "-write center.X" {
        w852 = cursor_action."write"  # action
        n308 = Unbundle By Name(w844) -> ("Plot ref"=w845:refnum<vi>, "cursors"=w851:i32[], "center"=w842:dbl)
        n309 = Index Array(array=w851, index #1=0 ("cursor index"), index #2=1 ("cursor index"), index #3=2 ("cursor index")) -> (element #2=w843:i32)  [unwired: 2 out]
        n310 = call "replace cursor - plot ref - V2.vi"("Plot ref in"=w845, "new X"=w842, "cursor index"=w843, "cursor action"=w852) -> ()  [unwired: 12 in, 4 out]
      }
      frame "-write center.Y" {
        w864 = cursor_action."write"  # action
        n311 = Unbundle By Name(w857) -> ("Plot ref"=w858:refnum<vi>, "cursors"=w863:i32[])
        n312 = Index Array(array=w863, index #1=0 ("cursor index"), index #2=1 ("cursor index"), index #3=2 ("cursor index")) -> (element #2=w854:i32)  [unwired: 2 out]
        n313 = Unbundle By Name(w856) -> ("center.Y"=w855:dbl)
        n314 = call "replace cursor - plot ref - V2.vi"("Plot ref in"=w858, "new  Y"=w855, "cursor index"=w854, "cursor action"=w864) -> ()  [unwired: 12 in, 4 out]
      }
      frame "-read all cursors" {
        w886 = cursor_action."read"  # action
        n315 = Unbundle By Name(w866) -> ("Plot ref"=w867:refnum<vi>, "cursors"=w884:i32[])
        n316 = Index Array(array=w884, index #1=0 ("cursor index"), index #2=1 ("cursor index"), index #3=2 ("cursor index")) -> (element #1=w885:i32, element #2=w881:i32, element #3=w879:i32)
        n317 = call "replace cursor - plot ref - V2.vi"("Plot ref in"=w867, "cursor index"=w885, "cursor action"=w886) -> ("Plot ref out"=w878:refnum<vi>, "read X"=w874:dbl, "read Y"=w873:dbl)  [unwired: 13 in, 1 out]
        n318 = call "replace cursor - plot ref - V2.vi"("Plot ref in"=w878, "cursor index"=w881, "cursor action"=w886) -> ("Plot ref out"=w877:refnum<vi>, "read X"=w872:dbl, "read Y"=w871:dbl)  [unwired: 13 in, 1 out]
        n319 = call "replace cursor - plot ref - V2.vi"("Plot ref in"=w877, "cursor index"=w879, "cursor action"=w886) -> ("read X"=w870:dbl, "read Y"=w869:dbl)  [unwired: 13 in, 2 out]
        n320 = Bundle By Name(cluster=w876, "left.X"=w874, "left.Y"=w873, "center.X"=w872, "center.Y"=w871, "right.X"=w870, "right.Y"=w869) -> (w875:T4)
      }
      frame "read" {
      }
      frame "-read cursor 2" {
        w904 = cursor_action."read"  # action
        n321 = Unbundle By Name(w893) -> ("Plot ref"=w894:refnum<vi>, "cursors"=w903:i32[])
        n322 = Index Array(array=w903, index #1=0 ("cursor index"), index #2=1 ("cursor index"), index #3=2 ("cursor index")) -> (element #3=w892:i32)  [unwired: 2 out]
        n323 = call "replace cursor - plot ref - V2.vi"("Plot ref in"=w894, "cursor index"=w892, "cursor action"=w904) -> ("read X"=w897:dbl, "read Y"=w896:dbl)  [unwired: 13 in, 2 out]
        n324 = Bundle By Name(cluster=w899, "right.X"=w897, "right.Y"=w896) -> (w898:T4)
      }
      frame "-read cursor 1" {
        w918 = cursor_action."read"  # action
        n325 = Unbundle By Name(w906) -> ("Plot ref"=w908:refnum<vi>, "cursors"=w917:i32[])
        n326 = Index Array(array=w917, index #1=0 ("cursor index"), index #2=1 ("cursor index"), index #3=2 ("cursor index")) -> (element #2=w907:i32)  [unwired: 2 out]
        n327 = call "replace cursor - plot ref - V2.vi"("Plot ref in"=w908, "cursor index"=w907, "cursor action"=w918) -> ("read X"=w911:dbl, "read Y"=w910:dbl)  [unwired: 13 in, 2 out]
        n328 = Bundle By Name(cluster=w913, "center.X"=w911, "center.Y"=w910) -> (w912:T4)
      }
      frame "-read cursor 0" {
        w932 = cursor_action."read"  # action
        n329 = Unbundle By Name(w920) -> ("Plot ref"=w922:refnum<vi>, "cursors"=w931:i32[])
        n330 = Index Array(array=w931, index #1=0 ("cursor index"), index #2=1 ("cursor index"), index #3=2 ("cursor index")) -> (element #1=w921:i32)  [unwired: 2 out]
        n331 = call "replace cursor - plot ref - V2.vi"("Plot ref in"=w922, "cursor index"=w921, "cursor action"=w932) -> ("read X"=w925:dbl, "read Y"=w924:dbl)  [unwired: 13 in, 2 out]
        n332 = Bundle By Name(cluster=w927, "left.X"=w925, "left.Y"=w924) -> (w926:T4)
      }
    }
    n333 = call "cursor window action stack.vi"("stack action"=stack_action_--_control."check", "command stack"=w28) -> ("stack is empty ?"=w26:bool, "command stack out"=w27:T3[])  [unwired: 7 in, 1 out]
  }
  "cursor window out" <- w11
  n334 = property class="Clust (strict)"(reference=w19, "Value"=w11) -> (reference out=→"cursor window out":refnum<vi>)  [unwired: 1 in, 1 out]
